vi "Swoish Grain Control.vi"() -> ()   [LabVIEW 2020]
uses:
  Type Defs/Motor Indicator.ctl
  Type Defs/Auto Params 1.ctl
  Type Defs/Numeric Big Up Down.ctl
  Type Defs/Auto Params 2.ctl
  Type Defs/Keyboard Button.ctl
  Type Defs/Email Config.ctl
  Type Defs/Alarm Limits.ctl
  Type Defs/Alarm Config.ctl
  Type Defs/PLC Coils.ctl
  Type Defs/Alarm Type.ctl
  <vilib>/Utility/miscctls.llb/LVPositionTypeDef.ctl
  Type Defs/Motor Pop-up Config Type Def.ctl
  Type Defs/Motors Type Def.ctl
  Type Defs/Motor Type Type Def.ctl
  Type Defs/Pop-up Corner Type Def.ctl
  Type Defs/Motor Data.ctl
  Type Defs/Info Config.ctl
  Type Defs/Modbus Mode.ctl
  Type Defs/HMI Coils.ctl
  Type Defs/Bin Indicator Type Def.ctl
  Type Defs/PLC Registers.ctl
  Type Defs/HMI Registers.ctl
  620634fb-1add-4c8b-beea-12df023673e0.vi
  142f28d0-f634-4b64-9fd9-03d418606ab8.vi
  <vilib>/httpClient/POSTBuffer.vi
  <vilib>/Comparison/Equal/Equal Functor/Equal Functor.lvclass
  <vilib>/httpClient/LabVIEWHTTPClient.lvlib
panel:
  in  "Array":u16[](array[slide])=[16055, 1251, 4170, 1460] scale=0.0..49000.0
  out "U-Trough":bool
  in  "Auto Mode Debug":bool
  in  "Exit":bool
  in  "Bin Levels Debug":u16[](array[numeric])
  out "Bin Levels":u16[](array[numeric])=[16055, 1251, 4170, 1460]
  in  "debug":bool
  in  "Alarms":T1[](array[typedef])=[{"PLC Coil"=enum."MC200_PLC_Estop_Main", "Alarm Type"=enum."Emergency", "Message"="The E-Stop on the main electrical enclosure was pushed.", "Shutdown"=TRUE, "Send Email"=TRUE}, {"PLC Coil"=enum."MC201_PLC_Estop_GSI", "Alarm Type"=enum."Emergency", "Message"="The E-Stop located on the GSI enclosure was pushed.", "Shutdown"=TRUE, "Send Email"=TRUE}, {"PLC Coil"=enum."MC202_PLC_Estop_Dryer", "Alarm Type"=enum."Emergency", "Message"="The E-Stop located at the Dryer was pushed.", "Shutdown"=TRUE, "Send Email"=TRUE}, {"PLC Coil"=enum."MC240_PLC_WS_Drag_OL", "Alarm Type"=enum."Warning", "Message"="Wet Silo Drag OVERLOAD.", "Shutdown"=FALSE, "Send Email"=TRUE}, {"PLC Coil"=enum."MC241_PLC_WB_Drag_OL", "Alarm Type"=enum."Warning", "Message"="Wet Bin Drag OVERLOAD.", "Shutdown"=FALSE, "Send Email"=TRUE}, {"PLC Coil"=enum."MC242_PLC_WS_Fan_OL", "Alarm Type"=enum."Warning", "Message"="Wet Silo Fan OVERLOAD.", "Shutdown"=FALSE, "Send Email"=TRUE}, {"PLC Coil"=enum."MC243_PLC_WB_Fan_OL", "Alarm Type"=enum."Warning", "Message"="Wet Bin Fan OVERLOAD.", "Shutdown"=FALSE, "Send Email"=TRUE}, {"PLC Coil"=enum."MC244_PLC_Dryr_Drag_OL", "Alarm Type"=enum."Warning", "Message"="Dryer Drag OVERLOAD.", "Shutdown"=FALSE, "Send Email"=TRUE}, {"PLC Coil"=enum."MC245_PLC_Dryr_Fan_OL", "Alarm Type"=enum."Warning", "Message"="Dryer Fan OVERLOAD.", "Shutdown"=FALSE, "Send Email"=TRUE}, {"PLC Coil"=enum."MC246_PLC_DB_Fan_Alm", "Alarm Type"=enum."Warning", "Message"="Dry Bin Fan VFD FAULT.", "Shutdown"=FALSE, "Send Email"=TRUE}, {"PLC Coil"=enum."MC247_PLC_DB_Drag_Alm", "Alarm Type"=enum."Warning", "Message"="Dry Bin Drag VFD FAULT.", "Shutdown"=FALSE, "Send Email"=TRUE}, {"PLC Coil"=enum."MC248_PLC_DB_Tp_Fd_Alm", "Alarm Type"=enum."Warning", "Message"="Dry Bin Top Feed VFD FAULT.", "Shutdown"=FALSE, "Send Email"=TRUE}, {"PLC Coil"=enum."MC249_PLC_U_Trough_Alm", "Alarm Type"=enum."Warning", "Message"="U-Trough VFD FAULT.", "Shutdown"=FALSE, "Send Email"=TRUE}, {"PLC Coil"=enum."MC250_PLC_Leg_Alm", "Alarm Type"=enum."Warning", "Message"="Leg VFD FAULT.", "Shutdown"=FALSE, "Send Email"=TRUE}, {"PLC Coil"=enum."MC261_PLC_Dryer_HI_Alm", "Alarm Type"=enum."Emergency", "Message"="The Dryer High Alarm limit switch has tripped.", "Shutdown"=TRUE, "Send Email"=TRUE}, {"PLC Coil"=enum."MC262_PLC_Dryr_Bin_Full", "Alarm Type"=enum."Warning", "Message"="The Dryer Bin Full limit switch has tripped.", "Shutdown"=FALSE, "Send Email"=TRUE}, {"PLC Coil"=enum."MC263_PLC_DB_HI_Alm", "Alarm Type"=enum."Warning", "Message"="The Dry Bin High Alarm limit switch has tripped.", "Shutdown"=FALSE, "Send Email"=TRUE}, {"PLC Coil"=enum."MC270_PLC_WS_Limit", "Alarm Type"=enum."Warning", "Message"="The Wet Silo has reached the level sensor limit.", "Shutdown"=FALSE, "Send Email"=TRUE}, {"PLC Coil"=enum."MC271_PLC_WB_Limit", "Alarm Type"=enum."Warning", "Message"="The Wet Bin has reached the level sensor limit.", "Shutdown"=FALSE, "Send Email"=TRUE}, {"PLC Coil"=enum."MC272_PLC_Dryr_Bin_Lim", "Alarm Type"=enum."Warning", "Message"="The Dryer Bin has reached the level sensor limit.", "Shutdown"=FALSE, "Send Email"=TRUE}, {"PLC Coil"=enum."MC273_PLC_DB_Limit", "Alarm Type"=enum."Warning", "Message"="The Dry Bin has reached the level sensor limit.", "Shutdown"=FALSE, "Send Email"=TRUE}, {"PLC Coil"=enum."MC274_PLC_Auto_Leg_Dry", "Alarm Type"=enum."Warning", "Message"="The Leg ran dry.  The Wet Bin or Silo may have run out of grain.", "Shutdown"=FALSE, "Send Email"=TRUE}, {"PLC Coil"=enum."MC280_Auto_Error_0", "Alarm Type"=enum."Warning", "Message"="While in Auto Mode, the Leg should have turned on, but didn't.", "Shutdown"=FALSE, "Send Email"=TRUE}, {"PLC Coil"=enum."MC281_Auto_Error_1", "Alarm Type"=enum."Warning", "Message"="While in Auto Mode, the Leg should have turned off, but didn't.", "Shutdown"=FALSE, "Send Email"=TRUE}, {"PLC Coil"=enum."MC282_Auto_Error_2", "Alarm Type"=enum."Warning", "Message"="While in Auto Mode, the Wet Bin Drag should have turned on, but didn't.", "Shutdown"=FALSE, "Send Email"=TRUE}, {"PLC Coil"=enum."MC283_Auto_Error_3", "Alarm Type"=enum."Warning", "Message"="While in Auto Mode, the Wet Bin Drag should have turned off, but didn't.", "Shutdown"=FALSE, "Send Email"=TRUE}, {"PLC Coil"=enum."MC284_Auto_Error_4", "Alarm Type"=enum."Warning", "Message"="While in Auto Mode, the Wet Silo Drag should have turned on, but didn't.", "Shutdown"=FALSE, "Send Email"=TRUE}, {"PLC Coil"=enum."MC285_Auto_Error_5", "Alarm Type"=enum."Warning", "Message"="While in Auto Mode, the Wet Silo Drag should have turned off, but didn't.", "Shutdown"=FALSE, "Send Email"=TRUE}, {"PLC Coil"=enum."MC286_Auto_Error_6", "Alarm Type"=enum."Warning", "Message"="While in Auto Mode, the Dry Bin Top Feed should have turned on, but didn't.", "Shutdown"=FALSE, "Send Email"=TRUE}, {"PLC Coil"=enum."MC287_Auto_Error_7", "Alarm Type"=enum."Warning", "Message"="While in Auto Mode, the Dry Bin Top Feed should have turned off, but didn't.", "Shutdown"=FALSE, "Send Email"=TRUE}]
  out "Heartbeat IN":bool
  out "Coils OUT":bool[](array[boolean])
  out "Registers OUT":u16[](array[numeric])
  out "Heartbeat OUT":bool=TRUE
  out "Loop Stop":bool
  out "PLC Disconnected":string="PLC DISCONNECTED!!!"
  in  "Alarm Pop-up":enum32{"Page 1"}(tab)
  in  "Alarm Ok PB":bool
  out "Alarm Title":string="Saturday, October 2, 2021  --  4:51:25 PM"
  out "Alarm Message":string="Saturday, October 2, 2021  --  4:51:25 PM"
  in  "VFD Pop-up":enum32{"Page 1"}(tab)
  in  "VFD_-1":bool
  in  "VFD_-0.1":bool
  in  "VFD_+0.1":bool
  in  "VFD_+1":bool
  out "VFD_Speed":dbl caption="bu" format="%.1f"
  out "VFD_Fault":bool caption="Fault"
  out "VFD_Running":bool caption="Running"
  in  "VFD_Toggle":bool
  in  "VFD_CMD":dbl caption="bu" min=0.0 max=60.0 format="%.1f"
  in  "VFD_Title":string="Leg"
  in  "Settings Pop-up":enum32{"Page 1"}(tab)
  in  "Settings Tab":T4(tab)=enum."Alarm Emails"
  in  "Auto Params 1":T5={"Leg Dry Limit:"=0, "Wet Drag Select:"=5, "Wet Drag Delay:"=0, "Leg Runout:"=0, "Dryer Bin Max:"=0, "Dryer Bin Min:"=0}
  in  "Auto Params 2":T7 {"Top Fd Auto Spd:" format="%.1f"}
  in  "Alarm Limits":T8={"Wet Silo Limit:"=5, "Wet Bin Limit:"=0, "Dryer Bin Limit:"=0, "Dry Bin Limit:"=0}
  in  "Email Config":T9[](array[typedef])=[{"Email"="garrett.tetil@gmail.com", "Enabled"=TRUE}, {"Email"="scott@myerselectricllc.com", "Enabled"=FALSE}, {"Email"="9896706221@txt.att.net", "Enabled"=TRUE}]
  in  "Settings Cancel PB":bool
  in  "Settings Ok PB":bool
  out "Auto Param Title":string="Settings"
  out "Keyboard PB":T10
  in  "Info Pop-up":enum32{"Page 1"}(tab)
  in  "Info Cancel PB":bool
  in  "Info Ok PB":bool
  out "Info Title":string="ATTENTION"
  out "Info Message":string="This will stop Auto Mode, and turn off all augers and drags."
  out "Motor_Sel (Round)":T11=TRUE
  out "Motor_Sel (Square)":bool
  in  "Motor Pop-up":enum32{"Page 1"}(tab)
  out "Motor_Overload":bool caption="Overload"
  out "Motor_Running":bool caption="Running"
  in  "Motor_Toggle":bool
  in  "Motor_Title":string="Wet Silo\nFan"
  in  "Main Tab":enum32{"Page 1"}(tab)
  in  "Reset Leg Dry PB":bool
  out "Leg Dry Run":bool
  out "DB Tp Fd Amps":dbl caption="bushel" format="%.1f A"
  out "Dryer Chute Open":bool
  out "Leg_Amps":dbl caption="bushel" format="%.1f A"
  out "Dryer Bin Level Limit":bool
  out "Wet Bin Level Limit":bool
  out "Wet Silo Level Limit":bool
  out "Dry Bin Level Limit":bool
  out "Auto Mode":bool
  in  "Settings PB":bool
  out "Date/Time String":string="Thursday, November 11, 2021  --  7:42:53 PM"
  out "Dryer Full":bool
  out "Dryer Bin Full":bool
  out "Dryer High Alarm":bool
  out "Dryer Feed":bool
  out "Dry Bin High Alarm":bool
  in  "Shutdown":bool
  in  "Auto/Manual PB":bool
  out "E-Stop (Dryer)":bool
  out "E-Stop (GSI)":bool
  out "E-Stop (Main)":bool
  out "WB_Numeric":u16=4170 caption="bushel"
  out "WS_Numeric":u16=1460 caption="bushel"
  out "Dryer_Numeric":u16=1251 caption="bushel"
  out "DB_Numeric":u16=16055 caption="bushel"
  out "DB_Scale":bool
  out "DB_Background":bool=TRUE
  out "DB_Fan":T11
  out "DB_Drag":T11
  out "Dryer_Fan":T11
  out "Dryer_Drag":T11
  out "WB_Fan":T11
  out "WS_Fan":T11
  out "WS_Drag":T11
  out "WB_Drag":T11
  out "Leg":bool
  out "DB_Top_Feed":bool
  out "Dryer_Scale":bool
  out "Dryer_Background":bool=TRUE
  out "WB_Scale":bool
  out "WB_Background":bool=TRUE
  out "WS_Scale":bool
  out "WS_Background":bool=TRUE
  # "Order dictates priority.\nMAKE VALUES DEFAULT!"
  # "Hz"
  # "Setpoint"
  # "Hz"
  # "Emails:"
  # "Enabled:"
  # "DRY BIN"
  # "WET SILO"
  # "DRY BIN\nTOP FEED"
  # "CONTROL\nROOM"
  # "LEG"
  # "DRYER /\nDRYER BIN"
  # "WET BIN"
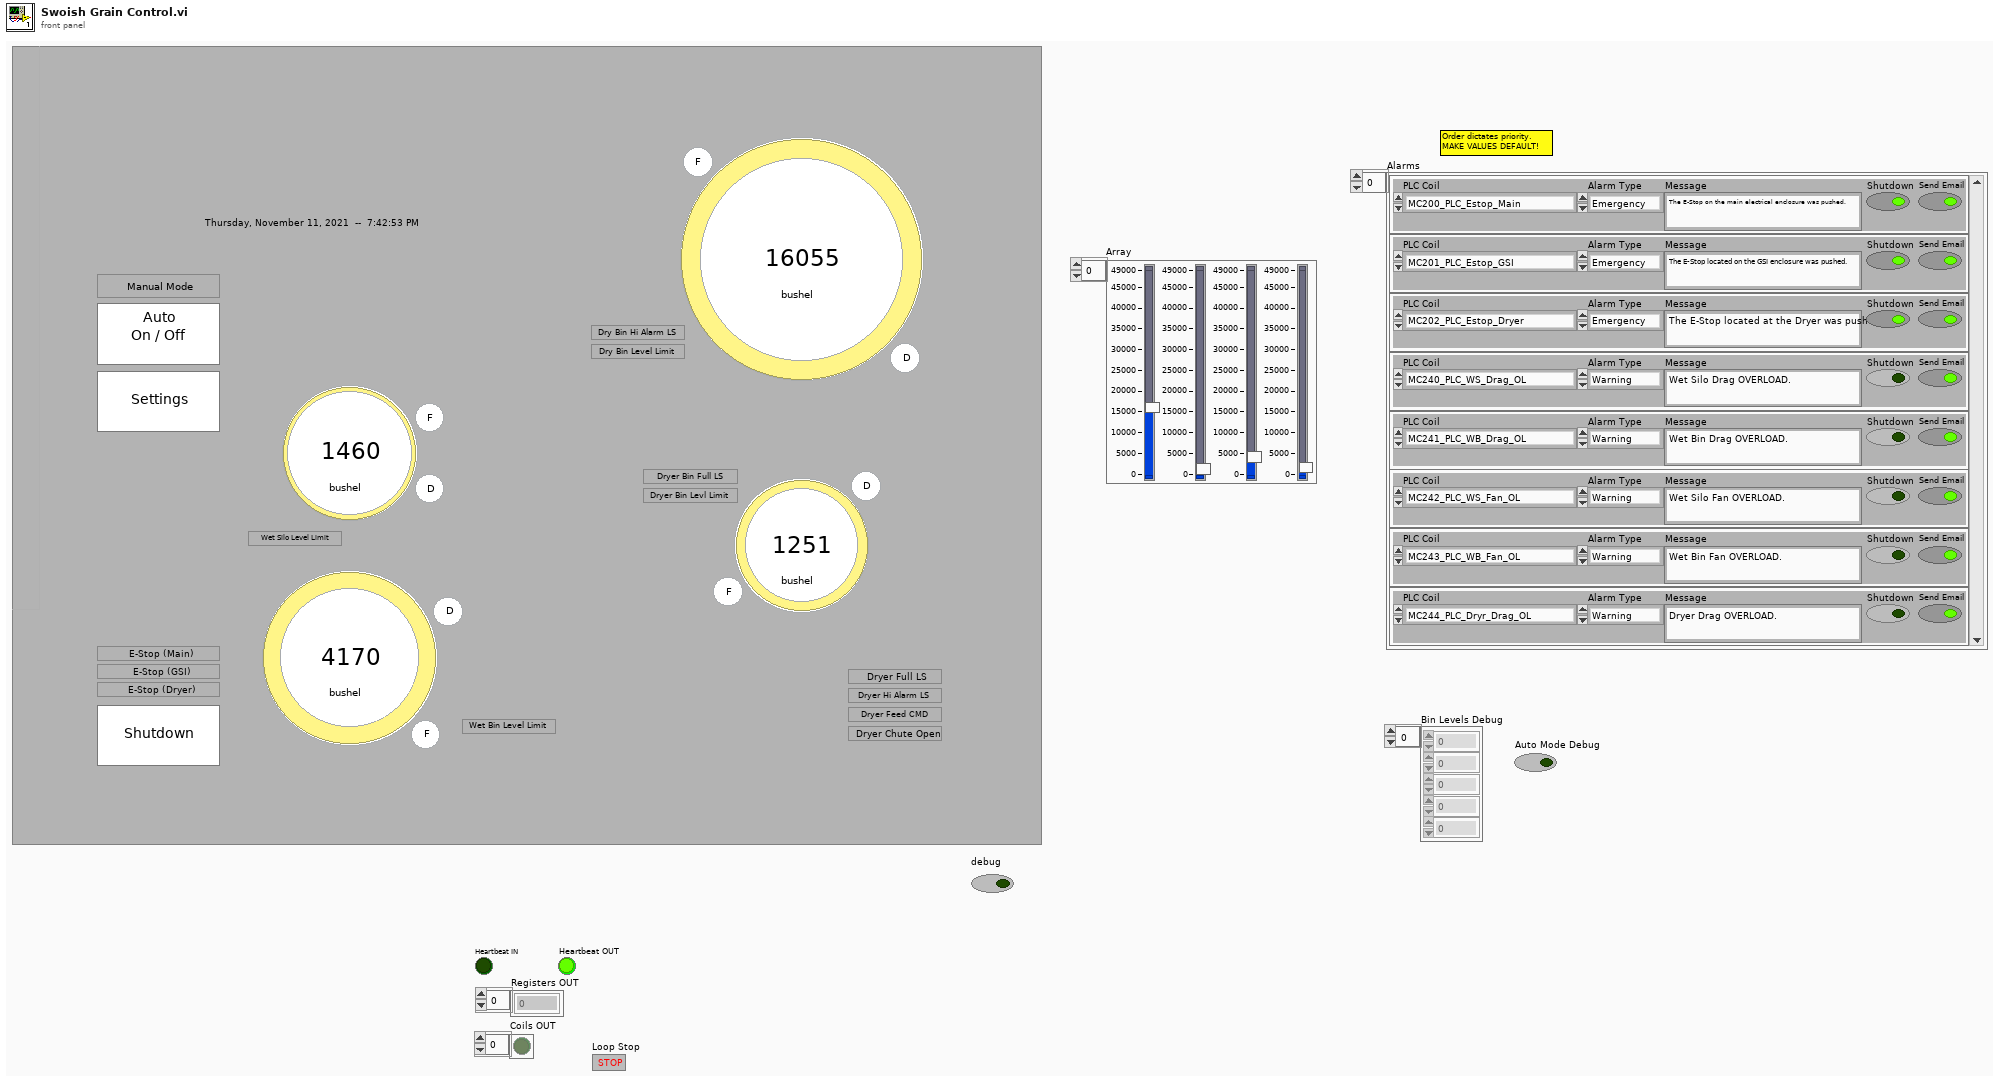
[diagram p1: front panel]
types:
  T1 = typedef "Alarm Config.ctl" = cluster{"PLC Coil":T2, "Alarm Type":T3, "Message":string, "Shutdown":bool, "Send Email":bool}
  T2 = typedef "PLC Coils.ctl" = enum16{"MC200_PLC_Estop_Main", "MC201_PLC_Estop_GSI", "MC202_PLC_Estop_Dryer", "MC203_PLC_Auto_Mode", "MC204", "MC205", "MC206", "MC207", "MC208", "MC209", "MC210", "MC211", "MC212", "MC213", "MC214", "MC215", "MC216", "MC217", "MC218", "MC219", "MC220_PLC_WS_Drag_ON", "MC221_PLC_WB_Drag_ON", "MC222_PLC_WS_Fan_ON", "MC223_PLC_WB_Fan_ON", "MC224_PLC_Dryr_Drag_ON", "MC225_PLC_Dryr_Fan_ON", "MC226", "MC227", "MC228", "MC229", "MC230", "MC231", "MC232", "MC233", "MC234", "MC235", "MC236", "MC237", "MC238", "MC239", "MC240_PLC_WS_Drag_OL", "MC241_PLC_WB_Drag_OL", "MC242_PLC_WS_Fan_OL", "MC243_PLC_WB_Fan_OL", "MC244_PLC_Dryr_Drag_OL", "MC245_PLC_Dryr_Fan_OL", "MC246_PLC_DB_Fan_Alm", "MC247_PLC_DB_Drag_Alm", "MC248_PLC_DB_Tp_Fd_Alm", "MC249_PLC_U_Trough_Alm", "MC250_PLC_Leg_Alm", "MC251", "MC252", "MC253", "MC254", "MC255", "MC256", "MC257", "MC258", "MC259", "MC260_PLC_Dryer_Full", "MC261_PLC_Dryer_HI_Alm", "MC262_PLC_Dryr_Bin_Full", "MC263_PLC_DB_HI_Alm", "MC264_PLC_Dryer_Chute", "MC265_PLC_Dryer_Feed", "MC266", "MC267", "MC268", "MC269", "MC270_PLC_WS_Limit", "MC271_PLC_WB_Limit", "MC272_PLC_Dryr_Bin_Lim", "MC273_PLC_DB_Limit", "MC274_PLC_Auto_Leg_Dry", "MC275", "MC276", "MC277", "MC278", "MC279", "MC280_Auto_Error_0", "MC281_Auto_Error_1", "MC282_Auto_Error_2", "MC283_Auto_Error_3", "MC284_Auto_Error_4", "MC285_Auto_Error_5", "MC286_Auto_Error_6", "MC287_Auto_Error_7", "MC288_Auto_Error_8", "MC289_Auto_Error_9"}
  T3 = typedef "Alarm Type.ctl" = enum16{"Warning", "Emergency"}
  T4 = enum32{"Auto Params", "Alarm Limits", "Alarm Emails"}
  T5 = typedef "Auto Params 1.ctl" = cluster{"Leg Dry Limit:":T6, "Wet Drag Select:":T6, "Wet Drag Delay:":T6, "Leg Runout:":T6, "Dryer Bin Max:":T6, "Dryer Bin Min:":T6}
  T6 = typedef "Numeric Big Up Down.ctl" = u16
  T7 = typedef "Auto Params 2.ctl" = cluster{"Top Fd Auto Spd:":dbl}
  T8 = typedef "Alarm Limits.ctl" = cluster{"Wet Silo Limit:":T6, "Wet Bin Limit:":T6, "Dryer Bin Limit:":T6, "Dry Bin Limit:":T6}
  T9 = typedef "Email Config.ctl" = cluster{"Email":string, "Enabled":bool}
  T10 = typedef "Keyboard Button.ctl" = bool
  T11 = typedef "Motor Indicator.ctl" = bool
  T12 = typedef "Info Config.ctl" = cluster{"Title":string, "Message":string, "Next State":string}
  T13 = typedef "Motor Data.ctl" = cluster{"Running":bool, "OL/Fault":bool, "VFD Speed":dbl, "VFD CMD":dbl}
  T14 = typedef "LVPositionTypeDef.ctl" = cluster{"Left":i32, "Top":i32}
  T15 = typedef "Motor Pop-up Config Type Def.ctl" = cluster{"Motor/VFD":T16, "Motor Type":T17, "Pop-up Corner":T18}
  T16 = typedef "Motors Type Def.ctl" = enum16{"WS_Drag", "WB_Drag", "WS_Fan", "WB_Fan", "Dryer_Drag", "Dryer_Fan", "DB_Fan", "DB_Drag", "DB_Top_Feed", "U-Trough", "Leg"}
  T17 = typedef "Motor Type Type Def.ctl" = enum16{"MS", "VFD"}
  T18 = typedef "Pop-up Corner Type Def.ctl" = enum16{"Top Left", "Top Right", "Bottom Left", "Bottom Right"}
  T19 = typedef "LabVIEWHTTPClient.lvlib/ClientHandle.ctl" = refnum<k1>
  T20 = cluster{"debug":bool, "Error":errorcluster, "Pop-up Config":T15, "Motor Descriptions":string[], "Pop-up Offset":T14, "Default Offset":T14, "Selected Motor Ref":refnum<vi>, "Motor Toggle":bool, "PLC Coils":bool[], "PLC Regs":u16[], "Motor Refs":refnum<vi>[], "Motor Data":T13[], "VFD_CMD":dbl, "Alarms":T1[], "Prev Alarm States":bool[], "Active Alarm Config":T1, "Active Alarm":bool, "Info Config":T12, "Params Open":bool, "Heartbeat Timer":u32, "Connected":bool, "Mode Toggle":bool, "Email Config":T9[], "Email Config Path":path}
  T21 = typedef "Modbus Mode.ctl" = enum16{"Init", "Read", "Write Coil", "Write Reg", "Param Read", "Param Write", "Close"}
  T22 = typedef "HMI Coils.ctl" = enum16{"MC100_HMI_WS_Drag_PB", "MC101_HMI_WB_Drag_PB", "MC102_HMI_WS_Fan_PB", "MC103_HMI_WB_Fan_PB", "MC104_HMI_Dryr_Drag_PB", "MC105_HMI_Dryr_Fan_PB", "MC106_HMI_DB_Fan_PB", "MC107_HMI_DB_Drag_PB", "MC108_HMI_DB_Top_Feed_PB", "MC109_HMI_U-Trough_PB", "MC110_HMI_Leg_PB", "MC111", "MC112", "MC113", "MC114", "MC115", "MC116", "MC117", "MC118", "MC119", "MC120_HMI_Shutdown", "MC121_HMI_Mode_Toggle", "MC122_HMI_Reset_Leg_Dry", "MC123"}
  T23 = cluster{"Running":bool, "OL/Fault":bool, "VFD Speed":dbl, "VFD CMD":dbl}
  T24 = typedef "Bin Indicator Type Def.ctl" = cluster{"Scale":refnum<vi>, "Background":refnum<vi>, "Numeric":refnum<vi>, "Bin Max":u16}
  T25 = enum8{"Enabled", "Disabled", "Disabled and Grayed Out"}
  T26 = typedef "PLC Registers.ctl" = enum16{"MHR200_PLC_DB_Fan_Spd", "MHR201_PLC_DB_Drag_Spd", "MHR202_PLC_DB_Tp_Fd_Spd", "MHR203_PLC_U_Trough_Spd", "MHR204_PLC_Leg_Spd", "MHR205_PLC_DB_Fan_ON", "MHR206_PLC_DB_Drag_ON", "MHR207_PLC_DB_Tp_Fd_ON", "MHR208_PLC_U_Trough_ON", "MHR209_PLC_Leg_ON", "MHR210_PLC_DB_Fan_CMD", "MHR211_PLC_DB_Drag_CMD", "MHR212_PLC_DB_Tp_Fd_CMD", "MHR213_PLC_U_Trough_CMD", "MHR214_PLC_Leg_CMD", "MHR215_PLC_DB_Fan_Flt", "MHR216_PLC_DB_Drag_Flt", "MHR217_PLC_DB_Tp_Fd_Flt", "MHR218_PLC_U_Trough_Flt", "MHR219_PLC_Leg_Flt", "MHR220_PLC_DB_Level", "MHR221_PLC_WB_Level", "MHR222_PLC_WS_Level", "MHR223_PLC_Dryr_Bin_Level", "MHR224_PLC_Leg_Amps", "MHR225_PLC_DB_Tp_Fd_Amps"}
  T27 = typedef "HMI Registers.ctl" = enum16{"MHR100_HMI_DB_Fan_CMD", "MHR101_HMI_DB_Drag_CMD", "MHR102_HMI_DB_TF_CMD", "MHR103_HMI_U_Trough_CMD", "MHR104_HMI_Leg_CMD"}
  T28 = cluster{"Running":bool, "OL/Fault":bool, "VFD Speed":dbl, "VFD CMD":dbl}[]
  T29 = cluster{"[0]":u16, "[1]":u16, "[2]":u16, "[3]":u16, "[4]":u16, "[5]":u16}
  T30 = cluster{"[0]":u16, "[1]":u16, "[2]":u16, "[3]":u16}
  T31 = enum32{"invalid app kind", "Development System", "Run Time System", "Student Edition", "Embedded LabVIEW", "Evaluation", "Custom"}
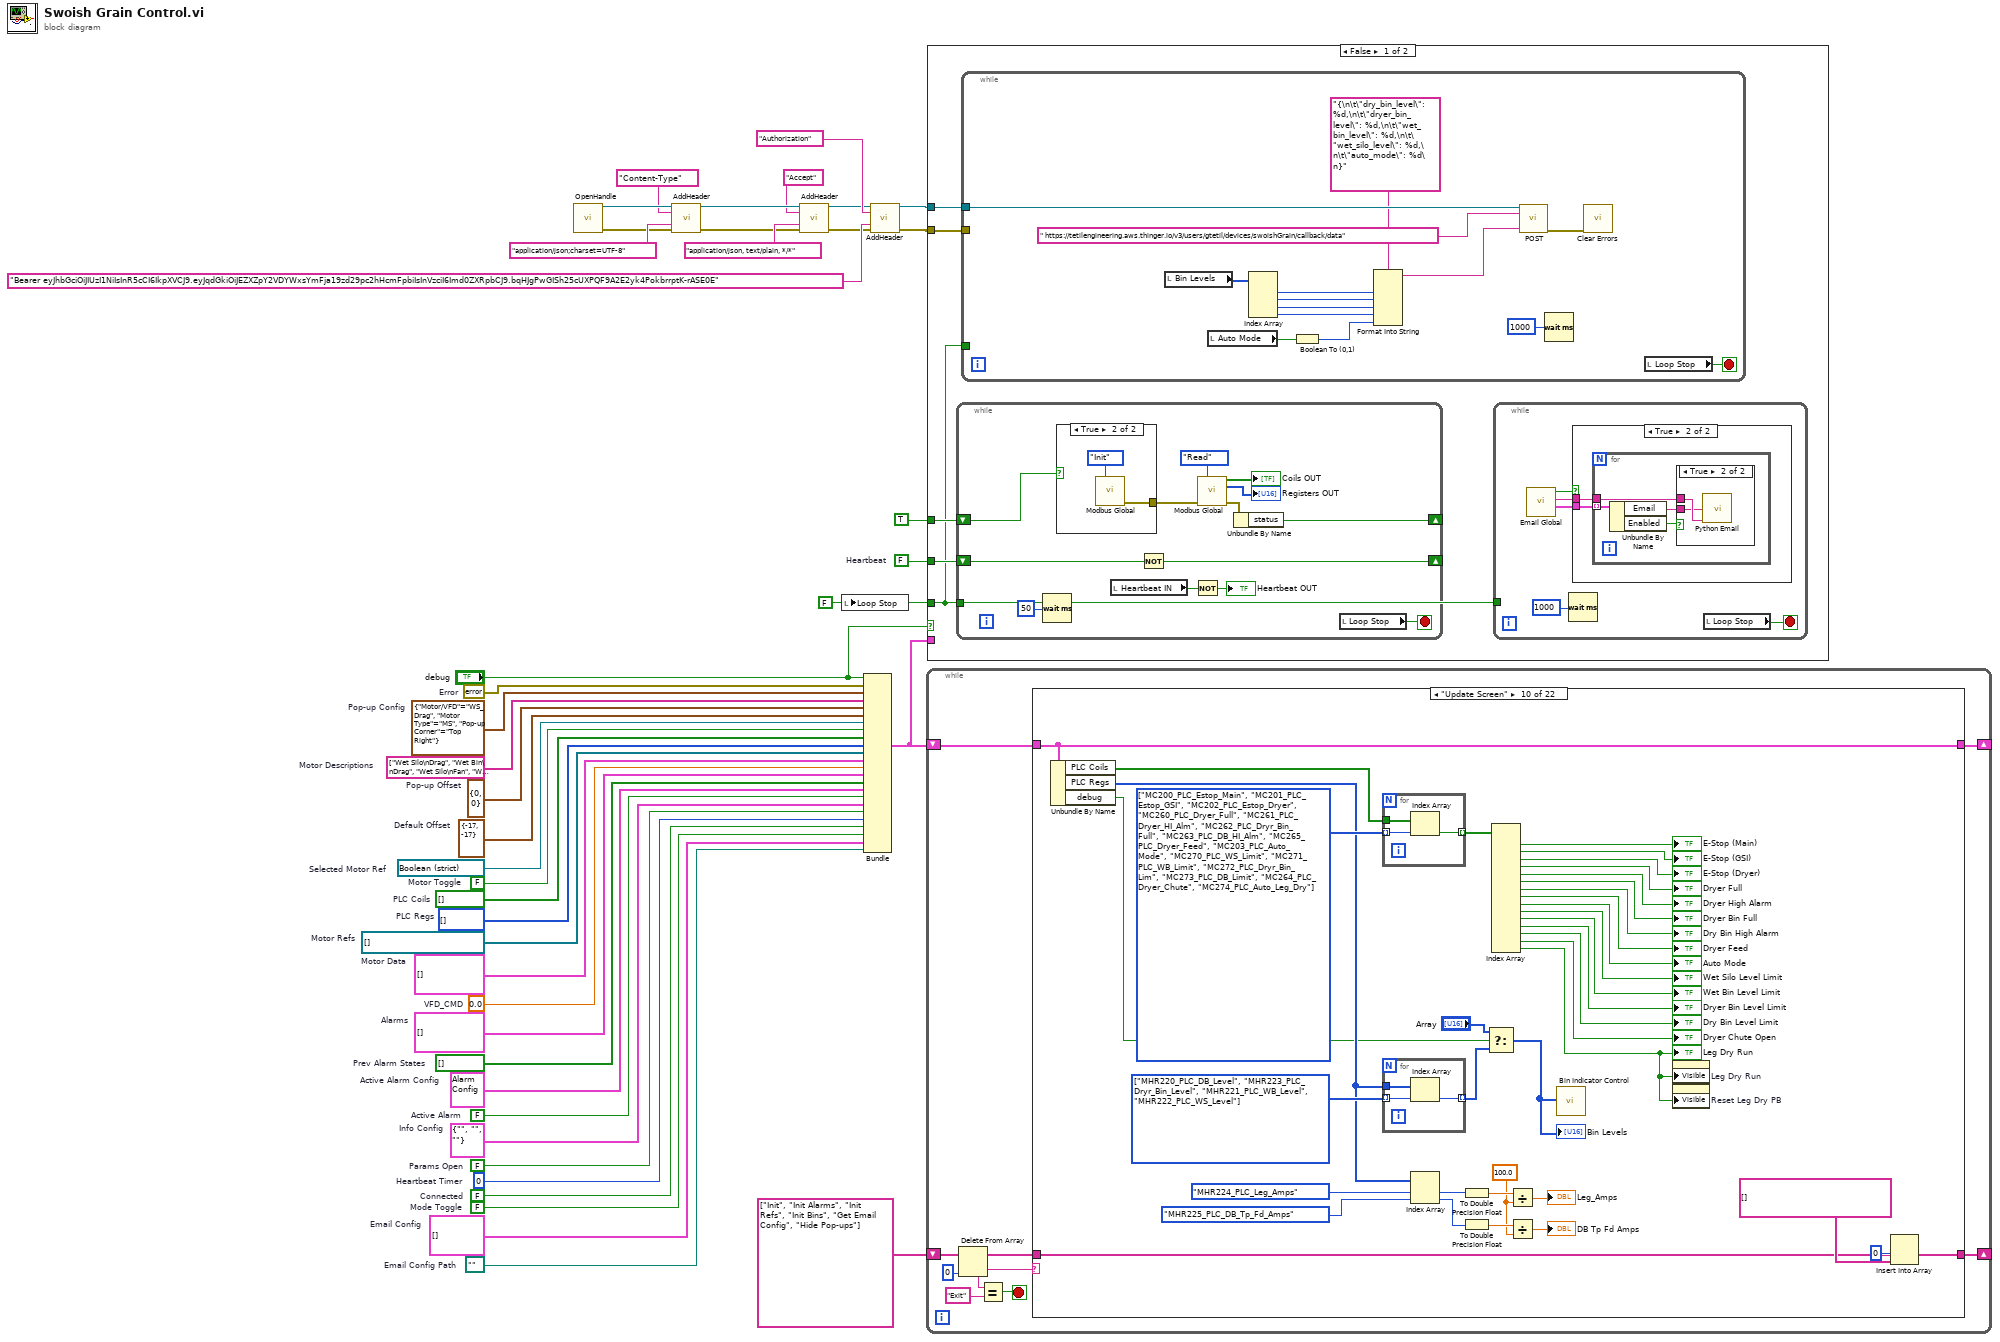
[diagram p0: block diagram]
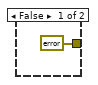
[diagram p2: hidden frame]
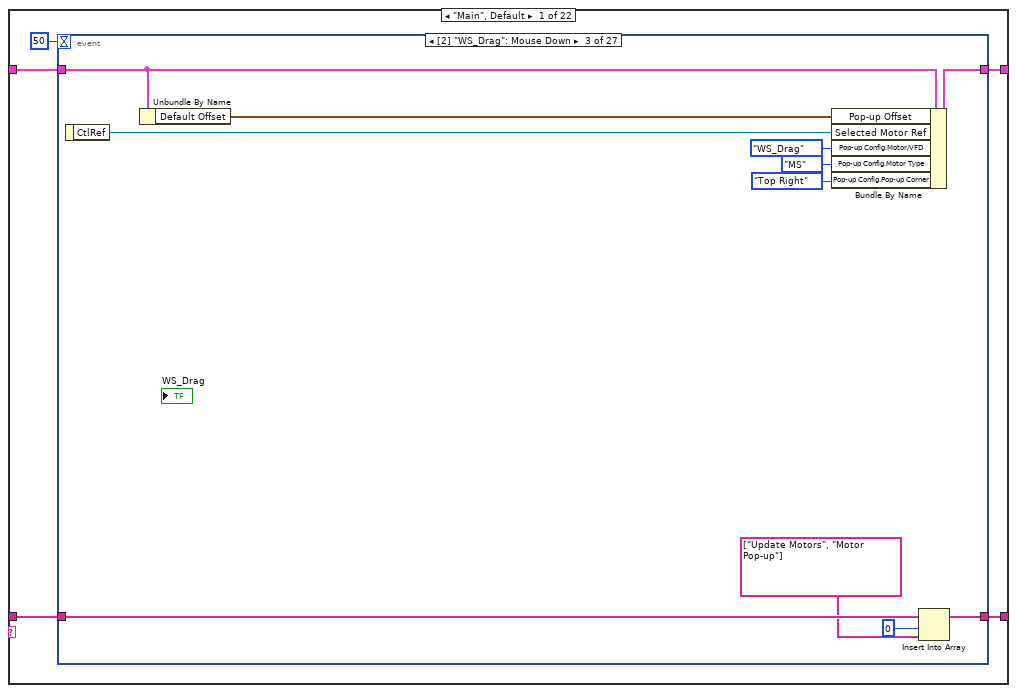
[diagram p6: hidden frame]
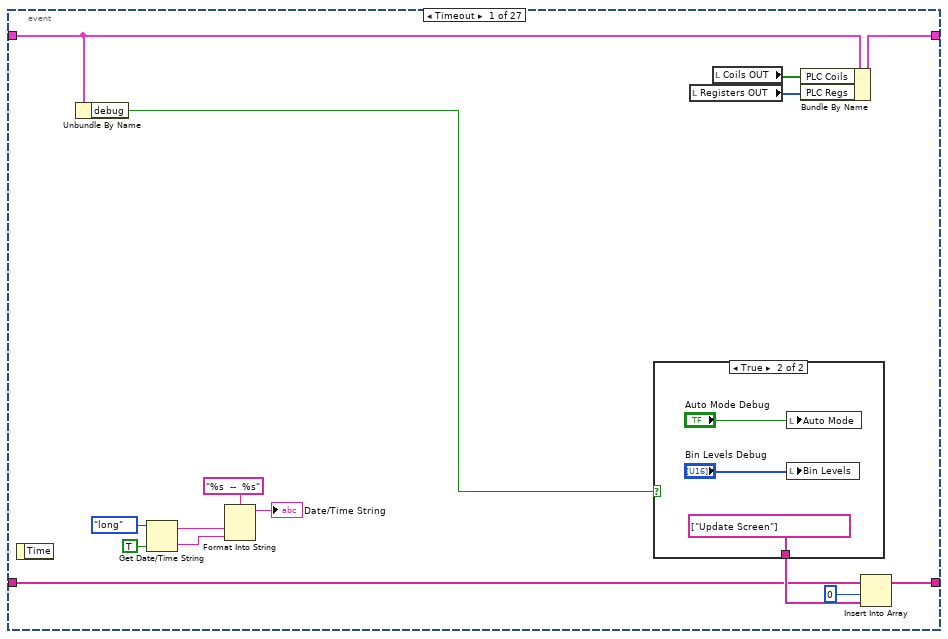
[diagram p7: hidden frame]
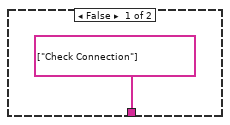
[diagram p8: hidden frame]
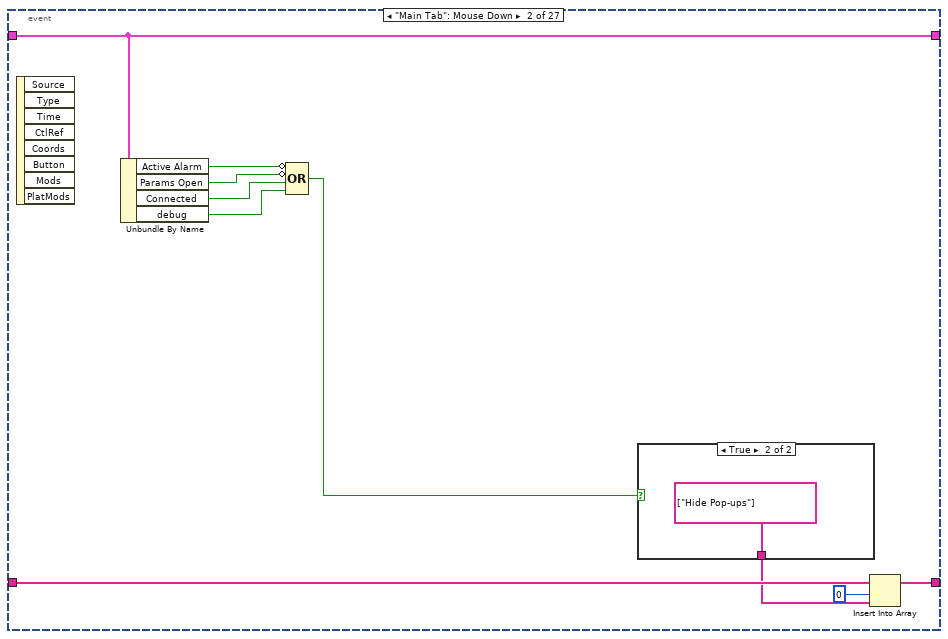
[diagram p9: hidden frame]
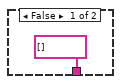
[diagram p10: hidden frame]
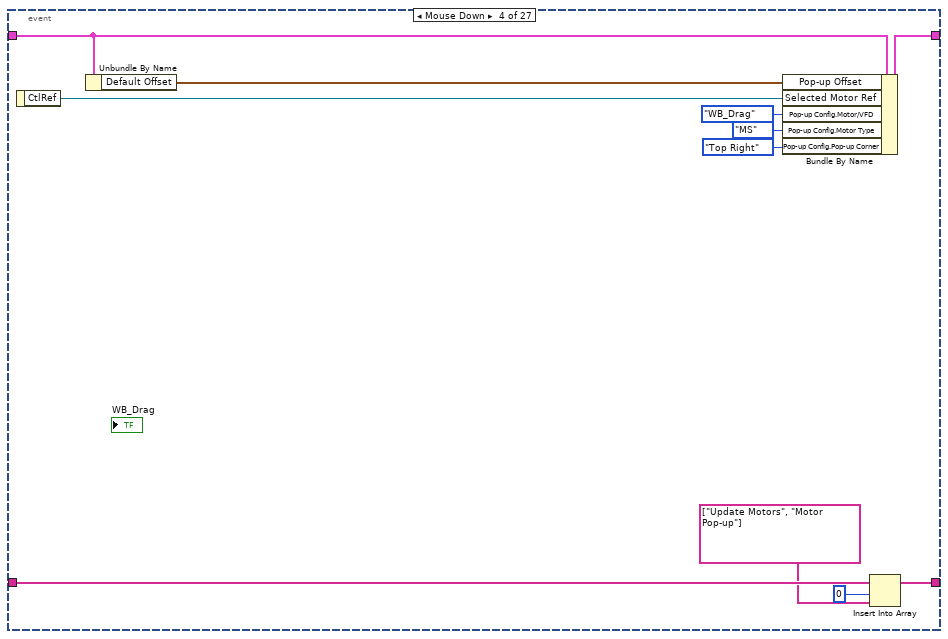
[diagram p11: hidden frame]
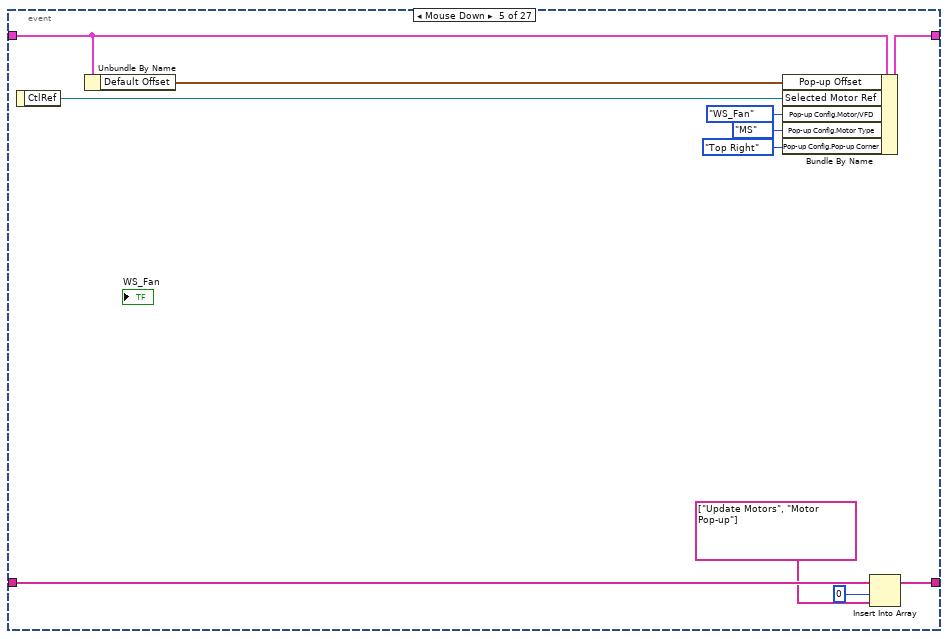
[diagram p12: hidden frame]
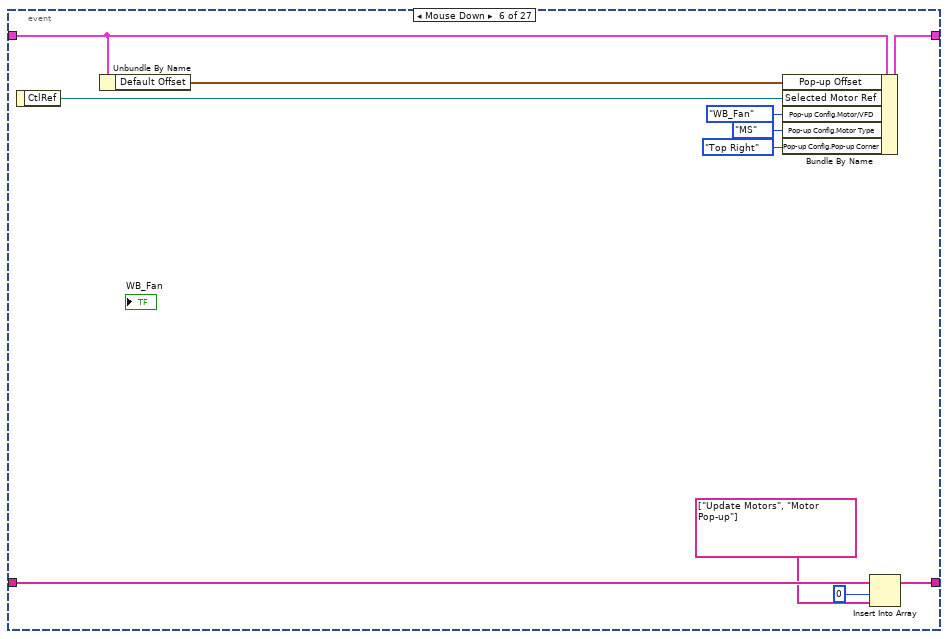
[diagram p13: hidden frame]
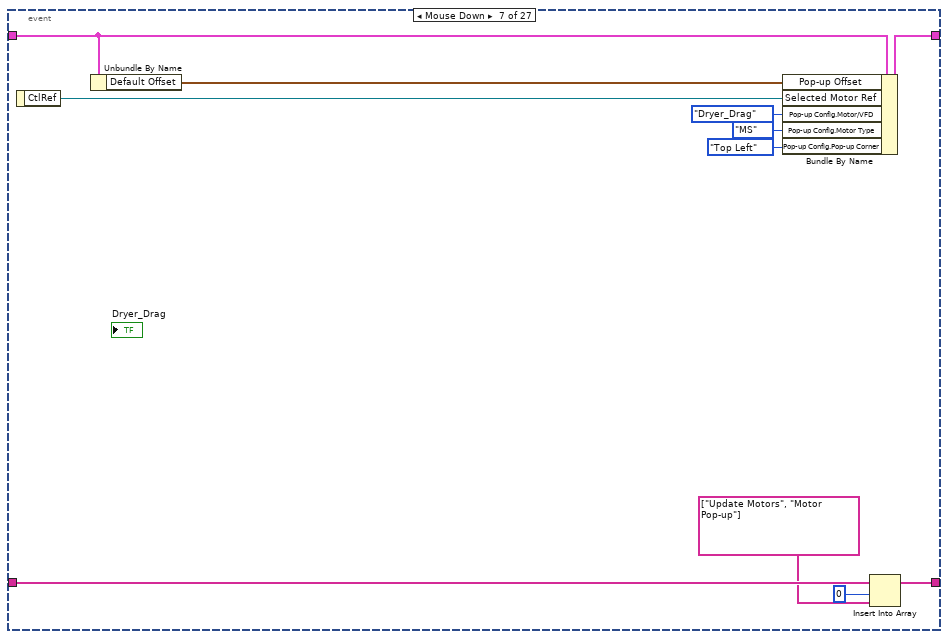
[diagram p14: hidden frame]
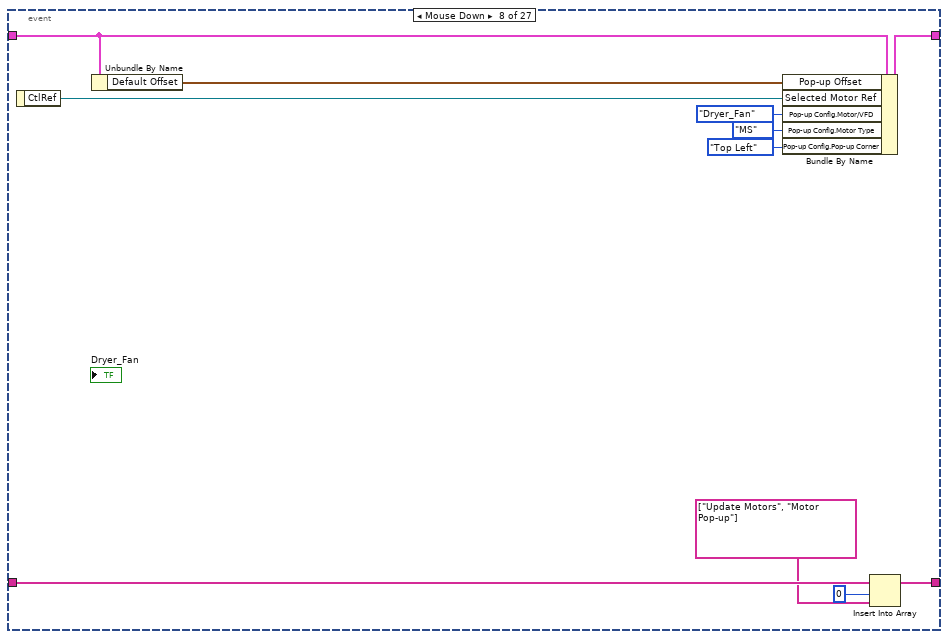
[diagram p15: hidden frame]
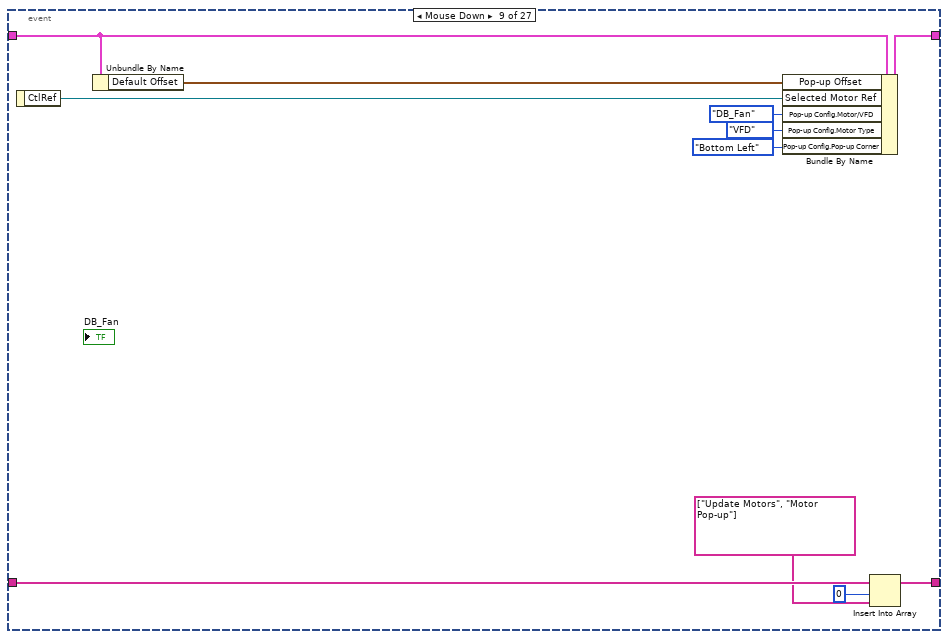
[diagram p16: hidden frame]
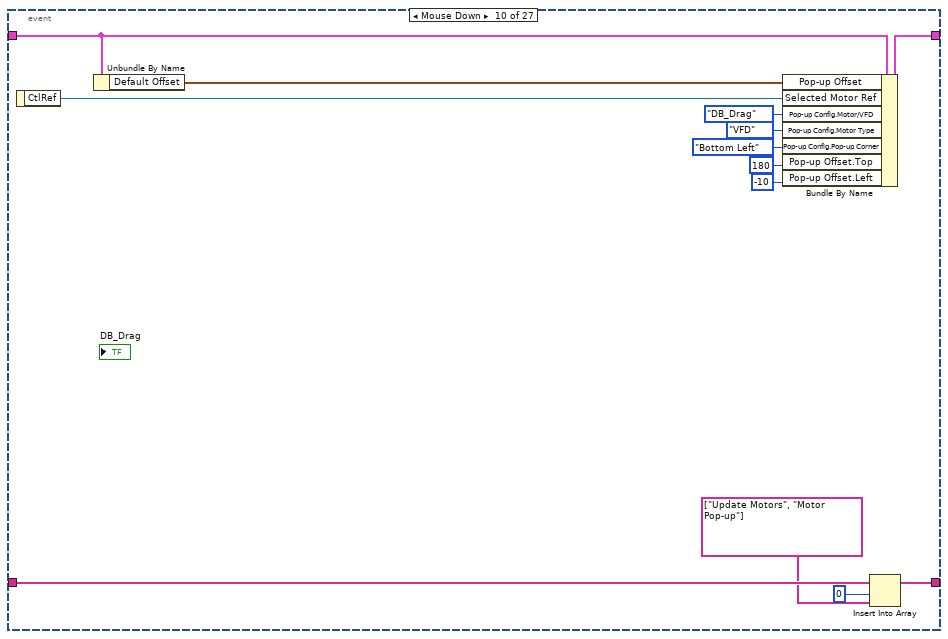
[diagram p17: hidden frame]
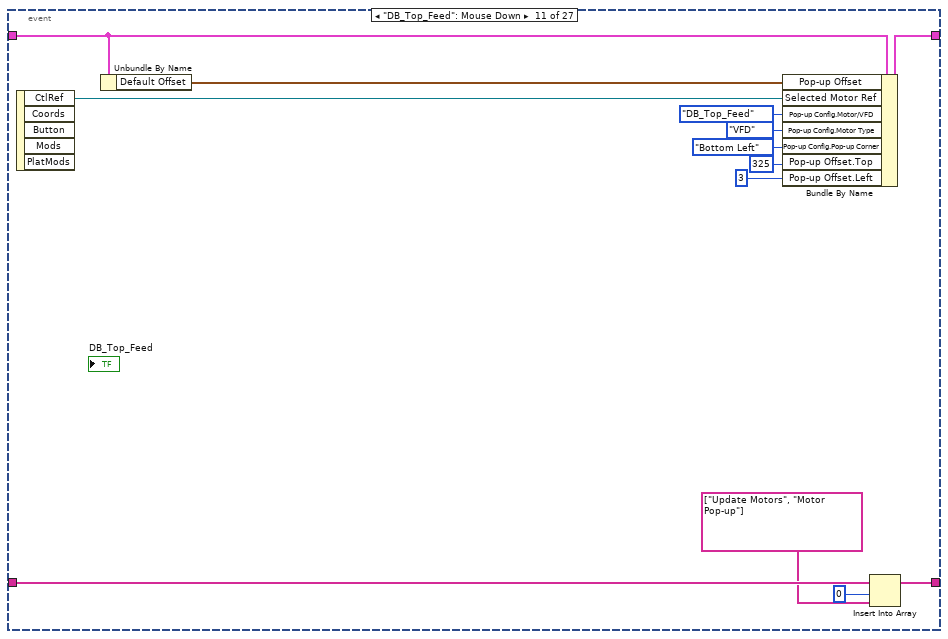
[diagram p18: hidden frame]
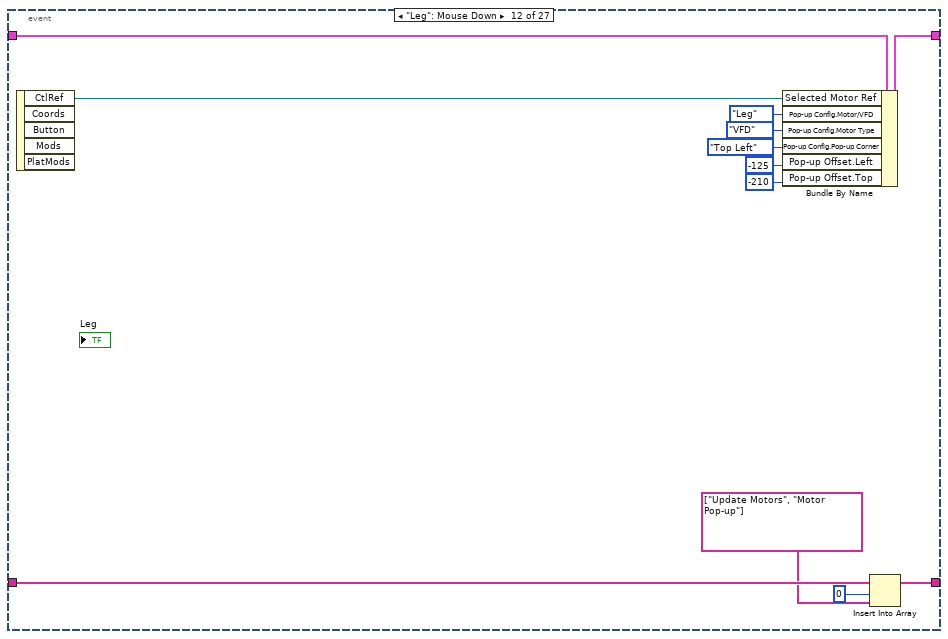
[diagram p19: hidden frame]
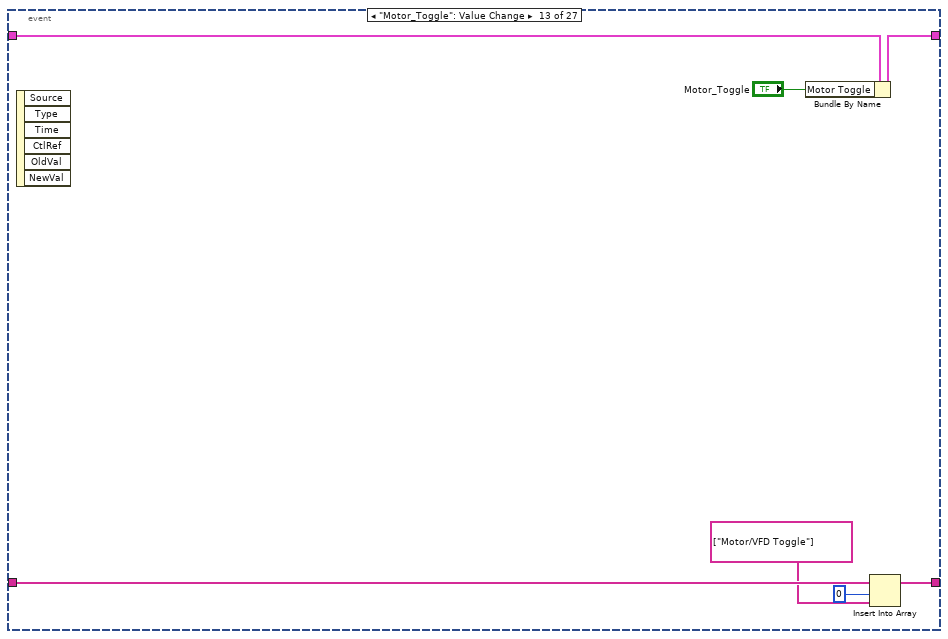
[diagram p20: hidden frame]
diagram:
  w18 = path ""  # Email Config Path
  w19 = T9[] []  # Email Config
  w20 = FALSE  # Mode Toggle
  w21 = FALSE  # Connected
  w23 = u32 0  # Heartbeat Timer
  w24 = FALSE  # Heartbeat
  w7 = FALSE ("Modbus Stop")
  w25 = FALSE  # Params Open
  w26 = T12 {"Title"="", "Message"="", "Next State"=""}  # Info Config
  w27 = FALSE  # Active Alarm
  w28 = T1 {"PLC Coil"=enum."MC200_PLC_Estop_Main", "Alarm Type"=enum."Warning", "Message"="", "Shutdown"=FALSE, "Send Email"=FALSE}  # Active Alarm Config
  w29 = bool[] []  # Prev Alarm States
  w30 = T1[] []  # Alarms
  w31 = 0.0  # VFD_CMD
  w32 = T13[] []  # Motor Data
  w33 = refnum<vi>[] []  # Motor Refs
  w34 = u16[] []  # PLC Regs
  w35 = bool[] []  # PLC Coils
  w36 = FALSE  # Motor Toggle
  w37 = T14 {"Left"=-17, "Top"=-17}  # Default Offset
  w38 = refnum<vi> refnum  # Selected Motor Ref
  w39 = T15 {"Motor/VFD"=enum."WS_Drag", "Motor Type"=enum."MS", "Pop-up Corner"=enum."Top Right"}  # Pop-up Config
  w41 = string[] ["Wet Silo\nDrag", "Wet Bin\nDrag", "Wet Silo\nFan", "Wet Bin\nFan", "Dryer\nDrag", "Dryer\nFan", "Dry Bin\nFan", "Dry Bin\nDrag", "Dry Bin\nTop Feed", "U-Trough", "Leg"]  # Motor Descriptions
  w40 = T14 {"Left"=0, "Top"=0}  # Pop-up Offset
  w42 = errorcluster {"status"=FALSE, "code"=0, "source"=""}  # Error
  n1 = call <vilib>:"OpenHandle.vi"() -> ("client handle out"=w17:T19, "error out"=w6:errorcluster)  [unwired: 14 in]
  n2 = call <vilib>:"AddHeader.vi"("client handle"=w17, "header"="Content-Type", "value"="application/json;charset=UTF-8", "error in (no error)"=w6) -> ("client handle out"=w11:T19, "error out"=w5:errorcluster)  [unwired: 10 in]
  n3 = call <vilib>:"AddHeader.vi"("client handle"=w11, "header"="Accept" ("value"), "value"="application/json, text/plain, */*", "error in (no error)"=w5) -> ("client handle out"=w10:T19, "error out"=w4:errorcluster)  [unwired: 10 in]
  n4 = local write "Loop Stop"(w7) -> ()
  n5 = Bundle("debug"="debug", "Error"=w42, "Pop-up Config"=w39, "Motor Descriptions"=w41, "Pop-up Offset"=w40, "Default Offset"=w37, "Selected Motor Ref"=w38, "Motor Toggle"=w36, "PLC Coils"=w35, "PLC Regs"=w34, "Motor Refs"=w33, "Motor Data"=w32, "VFD_CMD"=w31, "Alarms"=w30, "Prev Alarm States"=w29, "Active Alarm Config"=w28, "Active Alarm"=w27, "Info Config"=w26, "Params Open"=w25, "Heartbeat Timer"=w23, "Connected"=w21, "Mode Toggle"=w20, "Email Config"=w19, "Email Config Path"=w18) -> (w2:T20)  [unwired: 1 in]
  n6 = call <vilib>:"AddHeader.vi"("client handle"=w10, "header"="Authorization" ("value"), "value"="Bearer eyJhbGciOiJIUzI1NiIsInR5cCI6IkpXVCJ9.eyJqdGkiOiJEZXZpY2VDYWxsYmFja19zd29pc2hHcmFpbiIsInVzciI6Imd0ZXRpbCJ9.bqHJgPwGISh25cUXPQF9A2E2yk4PokbrrptK-rASE0E", "error in (no error)"=w4) -> ("client handle out"=w13:T19, "error out"=w3:errorcluster)  [unwired: 10 in]
  n7 = while {
    shift-right: [w47] -> _
    shift-left: w2 -> [w52]
    shift-right: [w48] -> _
    shift-left: string[] ["Init", "Init Alarms", "Init Refs", "Init Bins", "Get Email Config", "Hide Pop-ups"] -> [w51]
    stop <- w44 stop-if-true
    n8 = Delete From Array(array=w51, index=0) -> (deleted portion=w46:string, array with subset deleted=w49:string[])  [unwired: 1 in]
    n9 = Equal?(x=w46, y="Exit") -> (x = y?=w44:bool)
    n10 = case shown="\"Update Screen\"" w46 {
      tunnel: w52 -> [w57 w348 w357 w378 w412 w420 w429 w442 w480 w533 w556 w597 w615 w620 w633 w672 w700 w711 w734 w753 w764 w771]
      tunnel: w49 -> [w55 w350 w360 w381 w414 w426 w431 w451 w492 w535 w559 w584 w617 w624 w637 w680 w705 w713 w736 w755 w766 w774]
      tunnel: [w54 w349 w359 w380 w413 w425 w430 w435 w491 w534 w558 w599 w616 w623 w636 w679 w704 w712 w735 w754 w765 w773] -> w48
      tunnel: [w56 w348 w358 w379 w412 w421 w429 w443 w481 w533 w557 w598 w615 w620 w635 w673 w703 w711 w734 w753 w764 w771] -> w47
      frame "Main", Default {
        n11 = event shown="[2] \"WS_Drag\": Mouse Down" {
          selector: _ -> [_ _ _ _ _ _ _ _ _ _ _ _ _ _ _ _ _ _ _ _ _ _ _ _ _ _ _]
          dyn-events: _ -> [_ _ _ _ _ _ _ _ _ _ _ _ _ _ _ _ _ _ _ _ _ _ _ _ _ _ _]
          timeout: 50 -> [_ _ _ _ _ _ _ _ _ _ _ _ _ _ _ _ _ _ _ _ _ _ _ _ _ _ _]
          tunnel: w57 -> [w59 w82 w90 w102 w113 w124 w135 w146 w157 w170 w182 w197 w206 w213 w223 w247 w256 w264 w271 w282 w287 w291 w296 w310 w325 w333 w340]
          tunnel: [w62 w82 w95 w107 w118 w129 w140 w151 w162 w175 w188 w200 w205 w212 w231 w248 w256 w265 w272 w282 w287 w291 w296 w311 w325 w333 w340] -> w56
          tunnel: w55 -> [w69 w86 w99 w110 w121 w132 w143 w154 w165 w178 w191 w203 w210 w217 w235 w252 w260 w269 w276 w280 w286 w295 w300 w324 w329 w337 w344]
          tunnel: [w72 w85 w98 w109 w120 w131 w142 w153 w164 w177 w190 w202 w209 w216 w234 w251 w259 w268 w275 w285 w290 w294 w299 w323 w328 w336 w343] -> w54
          event Timeout {
            n12 = event-data() -> ()  [unwired: 1 in, 1 out]
            n13 = Unbundle By Name(w59) -> ("debug"=w58:bool)
            n14 = Get Date/Time String(date format (0)=enum16{"short", "long", "abbreviated"}."long", want seconds? (F)=TRUE) -> (date string=w67:string, time string=w66:string)  [unwired: 1 in]
            n15 = Format Into String(format string="%s  --  %s", w67, w66) -> (resulting string=→"Date/Time String":string)  [unwired: 2 in, 1 out]
            n16 = case shown="True" w58 {
              tunnel: [string[] ["Check Connection"] string[] ["Update Screen"]] -> w70
              frame False {
              }
              frame True {
                n17 = local write "Auto Mode"("Auto Mode Debug") -> ()
                n18 = local write "Bin Levels"("Bin Levels Debug") -> ()
              }
            }
            n19 = local read "Registers OUT"() -> (w60:u16[])
            n20 = local read "Coils OUT"() -> (w61:bool[])
            n21 = Bundle By Name(cluster=w59, "PLC Coils"=w61, "PLC Regs"=w60) -> (w62:T20)
            n22 = Insert Into Array(array=w69, index=0, new element=w70) -> (w72:string[])
          }
          event "Main Tab": Mouse Down {
            n23 = event-data() -> ()  [unwired: 1 in, 8 out]
            n24 = Unbundle By Name(w82) -> ("Active Alarm"=w81:bool, "Params Open"=w80:bool, "Connected"=w78:bool, "debug"=w77:bool)
            n25 = Compound Arithmetic op=OR(invert w81, invert w80, w78, w77) -> (w79:bool)
            n26 = case shown="True" w79 {
              tunnel: [string[] [] string[] ["Hide Pop-ups"]] -> w83
              frame False {
              }
              frame True {
              }
            }
            n27 = Insert Into Array(array=w86, index=0, new element=w83) -> (w85:string[])
          }
          event Mouse Down {
            n28 = event-data() -> ("CtlRef"=w91:refnum<vi>)  [unwired: 1 in]
            n29 = Unbundle By Name(w90) -> ("Default Offset"=w89:T14)
            n30 = Bundle By Name(cluster=w90, "Pop-up Offset"=w89, "Selected Motor Ref"=w91, "Pop-up Config.Motor/VFD"=Motors_Type_Def."WS_Drag" ("Pop-up Config.Motor"), "Pop-up Config.Motor Type"=Motor_Type_Type_Def."MS", "Pop-up Config.Pop-up Corner"=Pop-up_Corner_Type_Def."Top Right") -> (w95:T20)
            n31 = Insert Into Array(array=w99, index=0, new element=string[] ["Update Motors", "Motor Pop-up"]) -> (w98:string[])
          }
          event Mouse Down {
            n32 = event-data() -> ("CtlRef"=w103:refnum<vi>)  [unwired: 1 in]
            n33 = Unbundle By Name(w102) -> ("Default Offset"=w101:T14)
            n34 = Bundle By Name(cluster=w102, "Pop-up Offset"=w101, "Selected Motor Ref"=w103, "Pop-up Config.Motor/VFD"=Motors_Type_Def."WB_Drag" ("Pop-up Config.Motor"), "Pop-up Config.Motor Type"=Motor_Type_Type_Def."MS", "Pop-up Config.Pop-up Corner"=Pop-up_Corner_Type_Def."Top Right") -> (w107:T20)
            n35 = Insert Into Array(array=w110, index=0, new element=string[] ["Update Motors", "Motor Pop-up"]) -> (w109:string[])
          }
          event Mouse Down {
            n36 = event-data() -> ("CtlRef"=w114:refnum<vi>)  [unwired: 1 in]
            n37 = Unbundle By Name(w113) -> ("Default Offset"=w112:T14)
            n38 = Bundle By Name(cluster=w113, "Pop-up Offset"=w112, "Selected Motor Ref"=w114, "Pop-up Config.Motor/VFD"=Motors_Type_Def."WS_Fan" ("Pop-up Config.Motor"), "Pop-up Config.Motor Type"=Motor_Type_Type_Def."MS", "Pop-up Config.Pop-up Corner"=Pop-up_Corner_Type_Def."Top Right") -> (w118:T20)
            n39 = Insert Into Array(array=w121, index=0, new element=string[] ["Update Motors", "Motor Pop-up"]) -> (w120:string[])
          }
          event Mouse Down {
            n40 = event-data() -> ("CtlRef"=w125:refnum<vi>)  [unwired: 1 in]
            n41 = Unbundle By Name(w124) -> ("Default Offset"=w123:T14)
            n42 = Bundle By Name(cluster=w124, "Pop-up Offset"=w123, "Selected Motor Ref"=w125, "Pop-up Config.Motor/VFD"=Motors_Type_Def."WB_Fan" ("Pop-up Config.Motor"), "Pop-up Config.Motor Type"=Motor_Type_Type_Def."MS", "Pop-up Config.Pop-up Corner"=Pop-up_Corner_Type_Def."Top Right") -> (w129:T20)
            n43 = Insert Into Array(array=w132, index=0, new element=string[] ["Update Motors", "Motor Pop-up"]) -> (w131:string[])
          }
          event Mouse Down {
            n44 = event-data() -> ("CtlRef"=w136:refnum<vi>)  [unwired: 1 in]
            n45 = Unbundle By Name(w135) -> ("Default Offset"=w134:T14)
            n46 = Bundle By Name(cluster=w135, "Pop-up Offset"=w134, "Selected Motor Ref"=w136, "Pop-up Config.Motor/VFD"=Motors_Type_Def."Dryer_Drag" ("Pop-up Config.Motor"), "Pop-up Config.Motor Type"=Motor_Type_Type_Def."MS", "Pop-up Config.Pop-up Corner"=Pop-up_Corner_Type_Def."Top Left") -> (w140:T20)
            n47 = Insert Into Array(array=w143, index=0, new element=string[] ["Update Motors", "Motor Pop-up"]) -> (w142:string[])
          }
          event Mouse Down {
            n48 = event-data() -> ("CtlRef"=w147:refnum<vi>)  [unwired: 1 in]
            n49 = Unbundle By Name(w146) -> ("Default Offset"=w145:T14)
            n50 = Bundle By Name(cluster=w146, "Pop-up Offset"=w145, "Selected Motor Ref"=w147, "Pop-up Config.Motor/VFD"=Motors_Type_Def."Dryer_Fan" ("Pop-up Config.Motor"), "Pop-up Config.Motor Type"=Motor_Type_Type_Def."MS", "Pop-up Config.Pop-up Corner"=Pop-up_Corner_Type_Def."Top Left") -> (w151:T20)
            n51 = Insert Into Array(array=w154, index=0, new element=string[] ["Update Motors", "Motor Pop-up"]) -> (w153:string[])
          }
          event Mouse Down {
            n52 = event-data() -> ("CtlRef"=w158:refnum<vi>)  [unwired: 1 in]
            n53 = Unbundle By Name(w157) -> ("Default Offset"=w156:T14)
            n54 = Bundle By Name(cluster=w157, "Pop-up Offset"=w156, "Selected Motor Ref"=w158, "Pop-up Config.Motor/VFD"=Motors_Type_Def."DB_Fan" ("Pop-up Config.Motor"), "Pop-up Config.Motor Type"=Motor_Type_Type_Def."VFD", "Pop-up Config.Pop-up Corner"=Pop-up_Corner_Type_Def."Bottom Left") -> (w162:T20)
            n55 = Insert Into Array(array=w165, index=0, new element=string[] ["Update Motors", "Motor Pop-up"]) -> (w164:string[])
          }
          event Mouse Down {
            n56 = event-data() -> ("CtlRef"=w171:refnum<vi>)  [unwired: 1 in]
            n57 = Unbundle By Name(w170) -> ("Default Offset"=w169:T14)
            n58 = Bundle By Name(cluster=w170, "Pop-up Offset"=w169, "Selected Motor Ref"=w171, "Pop-up Config.Motor/VFD"=Motors_Type_Def."DB_Drag" ("Pop-up Config.Motor"), "Pop-up Config.Motor Type"=Motor_Type_Type_Def."VFD", "Pop-up Config.Pop-up Corner"=Pop-up_Corner_Type_Def."Bottom Left", "Pop-up Offset.Top"=180, "Pop-up Offset.Left"=-10) -> (w175:T20)
            n59 = Insert Into Array(array=w178, index=0, new element=string[] ["Update Motors", "Motor Pop-up"]) -> (w177:string[])
          }
          event "DB_Top_Feed": Mouse Down {
            n60 = event-data() -> ("CtlRef"=w184:refnum<vi>)  [unwired: 1 in, 4 out]
            n61 = Unbundle By Name(w182) -> ("Default Offset"=w181:T14)
            n62 = Bundle By Name(cluster=w182, "Pop-up Offset"=w181, "Selected Motor Ref"=w184, "Pop-up Config.Motor/VFD"=Motors_Type_Def."DB_Top_Feed" ("Pop-up Config.Motor"), "Pop-up Config.Motor Type"=Motor_Type_Type_Def."VFD", "Pop-up Config.Pop-up Corner"=Pop-up_Corner_Type_Def."Bottom Left", "Pop-up Offset.Top"=325, "Pop-up Offset.Left"=3) -> (w188:T20)
            n63 = Insert Into Array(array=w191, index=0, new element=string[] ["Update Motors", "Motor Pop-up"]) -> (w190:string[])
          }
          event "Leg": Mouse Down {
            n64 = event-data() -> ("CtlRef"=w196:refnum<vi>)  [unwired: 1 in, 4 out]
            n65 = Bundle By Name(cluster=w197, "Selected Motor Ref"=w196, "Pop-up Config.Motor/VFD"=Motors_Type_Def."Leg" ("Pop-up Config.Motor"), "Pop-up Config.Motor Type"=Motor_Type_Type_Def."VFD", "Pop-up Config.Pop-up Corner"=Pop-up_Corner_Type_Def."Top Left", "Pop-up Offset.Left"=-125, "Pop-up Offset.Top"=-210) -> (w200:T20)
            n66 = Insert Into Array(array=w203, index=0, new element=string[] ["Update Motors", "Motor Pop-up"]) -> (w202:string[])
          }
          event "Motor_Toggle": Value Change {
            n67 = event-data() -> ()  [unwired: 1 in, 6 out]
            n68 = Bundle By Name(cluster=w206, "Motor Toggle"="Motor_Toggle") -> (w205:T20)
            n69 = Insert Into Array(array=w210, index=0, new element=string[] ["Motor/VFD Toggle"]) -> (w209:string[])
          }
          event "VFD_Toggle": Value Change {
            n70 = event-data() -> ()  [unwired: 1 in, 6 out]
            n71 = Bundle By Name(cluster=w213, "Motor Toggle"="VFD_Toggle") -> (w212:T20)
            n72 = Insert Into Array(array=w217, index=0, new element=string[] ["Motor/VFD Toggle"]) -> (w216:string[])
          }
          event "VFD_+1", "VFD_+0.1", "VFD_-0.1", "VFD_-1": Value Change {
            n73 = event-data() -> ()  [unwired: 1 in, 6 out]
            n74 = Unbundle By Name(w223) -> ("VFD_CMD"=w222:dbl)
            n75 = Build Array("VFD_+1", "VFD_+0.1", "VFD_-0.1", "VFD_-1") -> (w226:bool[])
            n76 = call "Search Unsorted 1D Array.vim"("element"=TRUE, "unsorted 1D array"=w226) -> ("index of element"=w224:i32)  [unwired: 9 in]
            n77 = case shown="3" w224 {
              tunnel: w222 -> [w237 w240 w243 w244]
              tunnel: [w236 w238 w241 w245] -> w221
              frame 0, Default {
                n78 = Increment(x=w237) -> (x+1=w236:dbl)
              }
              frame 1 {
                n79 = Add(x=w240, y=0.1) -> (x+y=w238:dbl)
              }
              frame 2 {
                n80 = Subtract(x=w243, y=0.1) -> (x-y=w241:dbl)
              }
              frame 3 {
                n81 = Decrement(x=w244) -> (x-1=w245:dbl)
              }
            }
            n82 = In Range and Coerce(upper limit=60.0, x=w221, lower limit=0.0) -> (coerced(x)=w220:dbl)  [unwired: 1 out]
            n83 = Bundle By Name(cluster=w223, "VFD_CMD"=w220) -> (w231:T20)
            n84 = Insert Into Array(array=w235, index=0, new element=string[] ["Send VFD CMD"]) -> (w234:string[])
          }
          event "VFD_CMD": Value Change {
            n85 = event-data() -> ()  [unwired: 1 in, 6 out]
            n86 = Bundle By Name(cluster=w247, "VFD_CMD"="VFD_CMD") -> (w248:T20)
            n87 = Insert Into Array(array=w252, index=0, new element=string[] ["Send VFD CMD"]) -> (w251:string[])
          }
          event "VFD_CMD": Mouse Down {
            n88 = event-data() -> ()  [unwired: 1 in, 8 out]
            n89 = property on="Settings Pop-up" class="TabCtl (strict)"("Position"=T14 {"Left"=-1073, "Top"=-150}) -> ()  [unwired: 2 in, 2 out]
            n90 = constructor class="Process"() -> (reference out=w255:refnum<k24>)  [unwired: 3 in, 2 out]
            n91 = invoke class="Process" method="Start"(reference=w255, "fileName"="C:\\Program Files\\Common Files\\Microsoft Shared\\Ink\\TabTip.exe") -> ()  [unwired: 2 in, 4 out]
            n92 = Insert Into Array(array=w260, index=0, new element=string[] []) -> (w259:string[])
          }
          event "Shutdown": Value Change {
            n93 = event-data() -> ()  [unwired: 1 in, 6 out]
            n94 = Bundle By Name(cluster=w264, "Info Config.Title"="ATTENTION", "Info Config.Message"="This will stop Auto Mode, and turn off all augers and drags.", "Info Config.Next State"="Shutdown") -> (w265:T20)
            n95 = Insert Into Array(array=w269, index=0, new element=string[] ["Info Pop-up"]) -> (w268:string[])
          }
          event "Auto/Manual PB": Value Change {
            n96 = event-data() -> ()  [unwired: 1 in, 6 out]
            n97 = Bundle By Name(cluster=w271, "Mode Toggle"="Auto/Manual PB") -> (w272:T20)
            n98 = Insert Into Array(array=w276, index=0, new element=string[] ["Mode Toggle"]) -> (w275:string[])
          }
          event "Info Ok PB": Value Change {
            n99 = event-data() -> ()  [unwired: 1 in, 6 out]
            n100 = Unbundle By Name(w282) -> ("Info Config.Next State"=w278:string)
            n101 = Build Array(w278) -> (w277:string[])
            n102 = Insert Into Array(array=w280, index=0, new element=w277) -> (w279:string[])
            n103 = Insert Into Array(array=w279, index=0, new element=string[] ["Hide Pop-ups"]) -> (w285:string[])
          }
          event "Info Cancel PB": Value Change {
            n104 = event-data() -> ()  [unwired: 1 in, 6 out]
            n105 = Insert Into Array(array=w286, index=0, new element=string[] ["Hide Pop-ups"]) -> (w290:string[])
          }
          event "Alarm Ok PB": Value Change {
            n106 = event-data() -> ()  [unwired: 1 in, 6 out]
            n107 = Insert Into Array(array=w295, index=0, new element=string[] ["Hide Pop-ups"]) -> (w294:string[])
          }
          event "Settings PB": Value Change {
            n108 = event-data() -> ()  [unwired: 1 in, 6 out]
            n109 = Insert Into Array(array=w300, index=0, new element=string[] ["Settings Pop-up"]) -> (w299:string[])
          }
          event "Settings Ok PB": Value Change {
            w304 = 0  # Leg Dry Limit
            n110 = event-data() -> ()  [unwired: 1 in, 6 out]
            n111 = Unbundle By Name(w310) -> ("Email Config Path"=w312:path)
            n112 = Write to Binary File(file (use dialog)=w312, data="Email Config") -> ()  [unwired: 4 in, 3 out]
            n113 = Unbundle By Name("Auto Params 2") -> ("Top Fd Auto Spd:"=w316:dbl)
            n114 = Cluster To Array(cluster="Auto Params 1") -> (array=w306:T6[])
            n115 = Cluster To Array(cluster="Alarm Limits") -> (array=w307:T6[])
            n116 = Delete From Array(array=w306, length=1, index=w304) -> (deleted portion=w302:T6[], array with subset deleted=w303:T6[])
            n117 = Index Array(array=w302) -> (element=w301:T6)  [unwired: 1 in]
            n118 = Multiply(x=w316, y=100.0) -> (x*y=w314:dbl)
            n119 = To Unsigned Word Integer(number=w314) -> (unsigned 16bit integer=w313:u16)
            n120 = Build Array (concatenate)(w303, w313, w307, w301) -> (w318:T6[])
            n121 = call "Modbus Global.vi"("Modbus Mode (Write Coil)"=Modbus_Mode."Param Write", "Params IN"=w318) -> ()  [unwired: 10 in, 4 out]
            n122 = Bundle By Name(cluster=w310, "Email Config"="Email Config") -> (w311:T20)
            n123 = Insert Into Array(array=w324, index=0, new element=string[] ["Hide Pop-ups"]) -> (w323:string[])
          }
          event "Settings Cancel PB": Value Change {
            n124 = event-data() -> ()  [unwired: 1 in, 6 out]
            n125 = Insert Into Array(array=w329, index=0, new element=string[] ["Hide Pop-ups"]) -> (w328:string[])
          }
          event "Reset Leg Dry PB": Value Change {
            n126 = event-data() -> ()  [unwired: 1 in, 6 out]
            n127 = call "Modbus Global.vi"("HMI Coil"=HMI_Coils."MC122_HMI_Reset_Leg_Dry", "Modbus Mode (Write Coil)"=Modbus_Mode."Write Coil", "Coil IN"=TRUE) -> ()  [unwired: 9 in, 4 out]
            n128 = Insert Into Array(array=w337, index=0, new element=string[] []) -> (w336:string[])
          }
          event "Exit": Mouse Down {
            n129 = event-data() -> ("Mods"=w339:cluster{"Double Click":bool, "Menu Key":bool})  [unwired: 1 in, 7 out]
            n130 = Unbundle By Name(w339) -> ("Double Click"=w338:bool)
            n131 = case shown="True" w338 {
              tunnel: [string[] [] string[] ["Exit"]] -> w341
              frame False {
              }
              frame True {
              }
            }
            n132 = Insert Into Array(array=w344, index=0, new element=w341) -> (w343:string[])
          }
        }
      }
      frame "Init" {
        n133 = local write "Exit"(FALSE ("Exit")) -> ()
        n134 = Insert Into Array(array=w350, index=0, new element=string[] []) -> (w349:string[])
      }
      frame "Init Alarms" {
        n135 = Array Size(array="Alarms") -> (size(s)=w354:i32)
        n136 = Initialize Array(FALSE, w354) -> (w353:bool[])
        n137 = Bundle By Name(cluster=w357, "Alarms"="Alarms", "Prev Alarm States"=w353) -> (w358:T20)
        n138 = Insert Into Array(array=w360, index=0, new element=string[] []) -> (w359:string[])
      }
      frame "Init Refs" {
        n139 = control-ref of="WS_Drag"() -> (w377:refnum<vi>)
        n140 = control-ref of="WB_Drag"() -> (w376:refnum<vi>)
        n141 = control-ref of="WS_Fan"() -> (w375:refnum<vi>)
        n142 = control-ref of="WB_Fan"() -> (w374:refnum<vi>)
        n143 = control-ref of="Dryer_Drag"() -> (w373:refnum<vi>)
        n144 = control-ref of="Dryer_Fan"() -> (w372:refnum<vi>)
        n145 = control-ref of="DB_Fan"() -> (w371:refnum<vi>)
        n146 = control-ref of="DB_Drag"() -> (w370:refnum<vi>)
        n147 = control-ref of="DB_Top_Feed"() -> (w369:refnum<vi>)
        n148 = control-ref of="U-Trough"() -> (w363:refnum<vi>)
        n149 = control-ref of="Leg"() -> (w368:refnum<vi>)
        n150 = Build Array(w377, w376, w375, w374, w373, w372, w371, w370, w369, w363, w368) -> (w367:refnum<vi>[])
        n151 = Array Size(array=w367) -> (size(s)=w366:i32)
        n152 = for {
          tunnel: w367 -> [w384] mode=indexing
          n153 = property class="Bool (strict)"(reference=w384, "Value"=FALSE) -> ()  [unwired: 1 in, 2 out]
        }
        n154 = Initialize Array(T23 {"Running"=FALSE, "OL/Fault"=FALSE, "VFD Speed"=0.0, "VFD CMD"=0.0} ("Motor Data"), w366) -> (w364:T28)
        n155 = Bundle By Name(cluster=w378, "Motor Refs"=w367, "Motor Data"=w364) -> (w379:T20)
        n156 = Insert Into Array(array=w381, index=0, new element=string[] []) -> (w380:string[])
      }
      frame "Init Bins" {
        n157 = control-ref of="DB_Scale"() -> (w403:refnum<vi>)
        n158 = control-ref of="DB_Background"() -> (w404:refnum<vi>)
        n159 = control-ref of="WB_Scale"() -> (w406:refnum<vi>)
        n160 = control-ref of="WB_Background"() -> (w407:refnum<vi>)
        n161 = control-ref of="WS_Scale"() -> (w411:refnum<vi>)
        n162 = control-ref of="WS_Background"() -> (w410:refnum<vi>)
        n163 = control-ref of="Dryer_Scale"() -> (w393:refnum<vi>)
        n164 = control-ref of="Dryer_Background"() -> (w392:refnum<vi>)
        n165 = control-ref of="DB_Numeric"() -> (w405:refnum<vi>)
        n166 = control-ref of="WB_Numeric"() -> (w408:refnum<vi>)
        n167 = control-ref of="WS_Numeric"() -> (w409:refnum<vi>)
        n168 = control-ref of="Dryer_Numeric"() -> (w391:refnum<vi>)
        n169 = Bundle By Name(cluster=T24 {"Scale"=refnum, "Background"=refnum, "Numeric"=refnum, "Bin Max"=0} ("Bin Indicator Refs"), "Scale"=w403, "Background"=w404, "Numeric"=w405, "Bin Max"=u16 49373) -> (w395:T24)
        n170 = Bundle By Name(cluster=T24 {"Scale"=refnum, "Background"=refnum, "Numeric"=refnum, "Bin Max"=0} ("Bin Indicator Refs"), "Scale"=w406, "Background"=w407, "Numeric"=w408, "Bin Max"=u16 11025) -> (w387:T24)
        n171 = Bundle By Name(cluster=T24 {"Scale"=refnum, "Background"=refnum, "Numeric"=refnum, "Bin Max"=0} ("Bin Indicator Refs"), "Scale"=w411, "Background"=w410, "Numeric"=w409, "Bin Max"=u16 8865) -> (w388:T24)
        n172 = Bundle By Name(cluster=T24 {"Scale"=refnum, "Background"=refnum, "Numeric"=refnum, "Bin Max"=0} ("Bin Indicator Refs"), "Scale"=w393, "Background"=w392, "Numeric"=w391, "Bin Max"=u16 4128) -> (w386:T24)
        n173 = Build Array(w395, w386, w387, w388) -> (w394:T24[])
        n174 = call "Bin Indicator Control.vi"("Bin Indicator Refs"=w394, "Init (F)"=TRUE) -> ()  [unwired: 14 in]
        n175 = Insert Into Array(array=w414, index=0, new element=string[] []) -> (w413:string[])
      }
      frame "Get Email Config" {
        n176 = Unbundle By Name(w420) -> ("Email Config"=w422:T9[])
        n177 = call <vilib>:"Application Directory.vi"() -> ("Application Directory"=w424:path)
        n178 = Build Path(base path=w424, name or relative path=path "Email Config") -> (appended path=w417:path)
        n179 = Read from Binary File(5:w422, 11:w417) -> (0:w418:errorcluster, 2:w419:T9[])  [unwired: 4 in, 2 out]
        n180 = call <vilib>:"Clear Errors.vi"("error in (no error)"=w418) -> ()  [unwired: 5 in, 2 out]
        n181 = Bundle By Name(cluster=w420, "Email Config Path"=w417, "Email Config"=w419) -> (w421:T20)
        n182 = Insert Into Array(array=w426, index=0, new element=string[] []) -> (w425:string[])
      }
      frame "Unused Items" {
        n183 = Insert Into Array(array=w431, index=0, new element=string[] []) -> (w430:string[])
      }
      frame "Check Connection" {
        n184 = Unbundle By Name(w442) -> ("Heartbeat Timer"=w448:u32, "Connected"=w445:bool)
        n185 = Tick Count (ms)() -> (millisecond timer value=w446:u32)
        n186 = Subtract(x=w446, y=w448) -> (x-y=w450:u32)
        n187 = Greater?(x=w450, y=u32 200) -> (0:w449:bool)
        n188 = case shown="False" w449 {
          tunnel: [w467 w469] -> w447
          tunnel: w448 -> [w467 _]
          tunnel: w446 -> [_ w469]
          tunnel: [w466 w470] -> w438
          tunnel: w445 -> [w466 _]
          frame False {
          }
          frame True {
            n189 = local read "Heartbeat OUT"() -> (w468:bool)
            "Heartbeat IN" <- w468
            n190 = feedback #1() -> (w471:bool)  [unwired: 1 in]
            n191 = feedback-in #1(w468) -> ()
            n192 = Not Equal?(x=w468, y=w471) -> (x != y?=w470:bool)
          }
        }
        n193 = feedback #2() -> (w440:bool)  [unwired: 1 in]
        n194 = feedback-in #2(w438) -> ()
        n195 = case shown="True" w438 {
          tunnel: [string[] [] string[] ["Update Motors", "Update Screen", "Check Alarms"]] -> w441
          frame False {
          }
          frame True {
          }
        }
        n196 = Not Equal?(x=w438, y=w440) -> (x != y?=w439:bool)
        n197 = case shown="True" w439 {
          tunnel: w438 -> [_ w458]
          tunnel: [string[] [] w456] -> w434
          frame False {
          }
          frame True {
            n198 = case shown="False" w458 {
              tunnel: [TRUE ("Visible") FALSE ("Visible")] -> w459
              tunnel: [T25."Disabled and Grayed Out" ("Disabled") T25."Enabled" ("Disabled")] -> w457
              tunnel: [string[] ["Hide Pop-ups"] string[] []] -> w456
              frame False {
              }
              frame True {
              }
            }
            n199 = property on="PLC Disconnected" class="Str"("Visible"=w459) -> ()  [unwired: 2 in, 2 out]
            n200 = property on="Main Tab" class="TabCtl (strict)"("DisabledEnum"=w457) -> ()  [unwired: 2 in, 2 out]
          }
        }
        n201 = Insert Into Array(array=w451, index=0, new element=w441) -> (w436:string[])
        n202 = Bundle By Name(cluster=w442, "Heartbeat Timer"=w447, "Connected"=w438) -> (w443:T20)
        n203 = Insert Into Array(array=w436, index=0, new element=w434) -> (w435:string[])
      }
      frame "Update Motors" {
        w472 = 8  # Top Feed
        w473 = 10  # Leg
        n204 = Unbundle By Name(w480) -> ("Pop-up Config.Motor Type"=w489:T17, "Pop-up Config.Motor/VFD"=w486:T16, "Motor Refs"=w490:refnum<vi>[], "PLC Coils"=w488:bool[], "PLC Regs"=w487:u16[], "Motor Data"=w479:T13[])
        n205 = call "Update Motors.vi"("VFD Refs"=w490, "PLC Coils"=w488, "PLC Regs"=w487, "Motor Data IN"=w479) -> ("Motor Data OUT"=w477:T28)  [unwired: 15 in]
        n206 = Index Array(array=w477, index=w486) -> (element=w485:T23)
        n207 = Index Array(array=w477, index #1=w472, index #2=w473) -> (element #1=w478:T23, element #2=w474:T23)
        n208 = Unbundle By Name(w485) -> ("Running"=w484:bool, "OL/Fault"=w483:bool, "VFD Speed"=w482:dbl)
        n209 = Unbundle By Name(w478) -> ("Running"=w476:bool)
        n210 = Unbundle By Name(w474) -> ("Running"=w475:bool)
        n211 = case shown="\"VFD\"" w489 {
          tunnel: w484 -> [w496 w499]
          tunnel: w483 -> [w495 w498]
          tunnel: w482 -> [_ w497]
          frame "MS", Default {
            "Motor_Running" <- w496
            "Motor_Overload" <- w495
          }
          frame "VFD" {
            "VFD_Running" <- w499
            "VFD_Fault" <- w498
            "VFD_Speed" <- w497
          }
        }
        n212 = property on="DB Tp Fd Amps" class="DigNum (strict)"("Visible"=w476) -> ()  [unwired: 2 in, 2 out]
        n213 = property on="Leg_Amps" class="DigNum (strict)"("Visible"=w475) -> ()  [unwired: 2 in, 2 out]
        n214 = Bundle By Name(cluster=w480, "Motor Data"=w477) -> (w481:T20)
        n215 = Insert Into Array(array=w492, index=0, new element=string[] []) -> (w491:string[])
      }
      frame "Update Screen" {
        w507 = 100.0 ("y")
        w526 = T26[] [enum."MHR220_PLC_DB_Level", enum."MHR223_PLC_Dryr_Bin_Level", enum."MHR221_PLC_WB_Level", enum."MHR222_PLC_WS_Level"] items=["MHR200_PLC_DB_Fan_Spd", "MHR201_PLC_DB_Drag_Spd", "MHR202_PLC_DB_Tp_Fd_Spd", "MHR203_PLC_U_Trough_Spd", "MHR204_PLC_Leg_Spd", "MHR205_PLC_DB_Fan_ON", "MHR206_PLC_DB_Drag_ON", "MHR207_PLC_DB_Tp_Fd_ON", "MHR208_PLC_U_Trough_ON", "MHR209_PLC_Leg_ON", "MHR210_PLC_DB_Fan_CMD", "MHR211_PLC_DB_Drag_CMD", "MHR212_PLC_DB_Tp_Fd_CMD", "MHR213_PLC_U_Trough_CMD", "MHR214_PLC_Leg_CMD", "MHR215_PLC_DB_Fan_Flt", "MHR216_PLC_DB_Drag_Flt", "MHR217_PLC_DB_Tp_Fd_Flt", "MHR218_PLC_U_Trough_Flt", "MHR219_PLC_Leg_Flt", "MHR220_PLC_DB_Level", "MHR221_PLC_WB_Level", "MHR222_PLC_WS_Level", "MHR223_PLC_Dryr_Bin_Level", "MHR224_PLC_Leg_Amps", "MHR225_PLC_DB_Tp_Fd_Amps"]
        w531 = T2[] [enum."MC200_PLC_Estop_Main", enum."MC201_PLC_Estop_GSI", enum."MC202_PLC_Estop_Dryer", enum."MC260_PLC_Dryer_Full", enum."MC261_PLC_Dryer_HI_Alm", enum."MC262_PLC_Dryr_Bin_Full", enum."MC263_PLC_DB_HI_Alm", enum."MC265_PLC_Dryer_Feed", enum."MC203_PLC_Auto_Mode", enum."MC270_PLC_WS_Limit", enum."MC271_PLC_WB_Limit", enum."MC272_PLC_Dryr_Bin_Lim", enum."MC273_PLC_DB_Limit", enum."MC264_PLC_Dryer_Chute", enum."MC274_PLC_Auto_Leg_Dry"] items=["MC200_PLC_Estop_Main", "MC201_PLC_Estop_GSI", "MC202_PLC_Estop_Dryer", "MC203_PLC_Auto_Mode", "MC204", "MC205", "MC206", "MC207", "MC208", "MC209", "MC210", "MC211", "MC212", "MC213", "MC214", "MC215", "MC216", "MC217", "MC218", "MC219", "MC220_PLC_WS_Drag_ON", "MC221_PLC_WB_Drag_ON", "MC222_PLC_WS_Fan_ON", "MC223_PLC_WB_Fan_ON", "MC224_PLC_Dryr_Drag_ON", "MC225_PLC_Dryr_Fan_ON", "MC226", "MC227", "MC228", "MC229", "MC230", "MC231", "MC232", "MC233", "MC234", "MC235", "MC236", "MC237", "MC238", "MC239", "MC240_PLC_WS_Drag_OL", "MC241_PLC_WB_Drag_OL", "MC242_PLC_WS_Fan_OL", "MC243_PLC_WB_Fan_OL", "MC244_PLC_Dryr_Drag_OL", "MC245_PLC_Dryr_Fan_OL", "MC246_PLC_DB_Fan_Alm", "MC247_PLC_DB_Drag_Alm", "MC248_PLC_DB_Tp_Fd_Alm", "MC249_PLC_U_Trough_Alm", "MC250_PLC_Leg_Alm", "MC251", "MC252", "MC253", "MC254", "MC255", "MC256", "MC257", "MC258", "MC259", "MC260_PLC_Dryer_Full", "MC261_PLC_Dryer_HI_Alm", "MC262_PLC_Dryr_Bin_Full", "MC263_PLC_DB_HI_Alm", "MC264_PLC_Dryer_Chute", "MC265_PLC_Dryer_Feed", "MC266", "MC267", "MC268", "MC269", "MC270_PLC_WS_Limit", "MC271_PLC_WB_Limit", "MC272_PLC_Dryr_Bin_Lim", "MC273_PLC_DB_Limit", "MC274_PLC_Auto_Leg_Dry", "MC275", "MC276", "MC277", "MC278", "MC279", "MC280_Auto_Error_0", "MC281_Auto_Error_1", "MC282_Auto_Error_2", "MC283_Auto_Error_3", "MC284_Auto_Error_4", "MC285_Auto_Error_5", "MC286_Auto_Error_6", "MC287_Auto_Error_7", "MC288_Auto_Error_8", "MC289_Auto_Error_9"]
        n216 = Unbundle By Name(w533) -> ("PLC Coils"=w532:bool[], "PLC Regs"=w515:u16[], "debug"=w503:bool)
        n217 = for {
          tunnel: w532 -> [w543]
          tunnel: w531 -> [w542] mode=indexing
          tunnel: [w541] -> w530 mode=indexing
          n218 = Index Array(array=w543, index=w542) -> (element=w541:bool)
        }
        n219 = for {
          tunnel: w515 -> [w540]
          tunnel: w526 -> [w539] mode=indexing
          tunnel: [w538] -> w502 mode=indexing
          n220 = Index Array(array=w540, index=w539) -> (element=w538:u16)
        }
        n221 = Index Array(array=w515, index #1=PLC_Registers."MHR224_PLC_Leg_Amps" ("PLC Reg"), index #2=PLC_Registers."MHR225_PLC_DB_Tp_Fd_Amps" ("PLC Reg")) -> (element #1=w513:u16, element #2=w506:u16)
        n222 = To Double Precision Float(number=w513) -> (double precision float=w512:dbl)
        n223 = To Double Precision Float(number=w506) -> (double precision float=w508:dbl)
        n224 = Select(t="Array", s=w503, f=w502) -> (s? t:f=w501:u16[])
        "Bin Levels" <- w501
        n225 = Index Array(array=w530) -> (element #1=→"E-Stop (Main)":bool, element #2=→"E-Stop (GSI)":bool, element #3=→"E-Stop (Dryer)":bool, element #4=→"Dryer Full":bool, element #5=→"Dryer High Alarm":bool, element #6=→"Dryer Bin Full":bool, element #7=→"Dry Bin High Alarm":bool, element #8=→"Dryer Feed":bool, element #9=→"Auto Mode":bool, element #10=→"Wet Silo Level Limit":bool, element #11=→"Wet Bin Level Limit":bool, element #12=→"Dryer Bin Level Limit":bool, element #13=→"Dry Bin Level Limit":bool, element #14=→"Dryer Chute Open":bool, element #15=w504:bool)  [unwired: 15 in]
        "Leg Dry Run" <- w504
        n226 = Divide(x=w512, y=w507) -> (x/y=→"Leg_Amps":dbl)
        n227 = Divide(x=w508, y=w507) -> (x/y=→"DB Tp Fd Amps":dbl)
        n228 = call "Bin Indicator Control.vi"("Bin Levels"=w501) -> ()  [unwired: 15 in]
        n229 = property on="Leg Dry Run" class="Bool (strict)"("Visible"=w504) -> ()  [unwired: 2 in, 2 out]
        n230 = property on="Reset Leg Dry PB" class="Bool (strict)"("Visible"=w504) -> ()  [unwired: 2 in, 2 out]
        n231 = Insert Into Array(array=w535, index=0, new element=string[] []) -> (w534:string[])
      }
      frame "Check Alarms" {
        n232 = Unbundle By Name(w556) -> ("PLC Coils"=w547:bool[], "Prev Alarm States"=w548:bool[], "Alarms"=w553:T1[], "Active Alarm Config"=w546:T1, "Active Alarm"=w550:bool, "Active Alarm Config.Alarm Type"=w552:T3)
        n233 = Equal?(x=w552, y=Alarm_Type."Emergency") -> (x = y?=w549:bool)
        n234 = for {
          tunnel: w547 -> [w576]
          tunnel: w553 -> [w575] mode=indexing
          tunnel: [w573] -> w544 mode=indexing
          n235 = Unbundle By Name(w575) -> ("PLC Coil"=w574:T2)
          n236 = Index Array(array=w576, index=w574) -> (element=w573:bool)
        }
        n237 = And(x=w550, y=w549) -> (x .and. y?=w545:bool)
        n238 = case shown="False" w545 {
          tunnel: [w566 w572] -> w555
          tunnel: [w565 FALSE] -> w554
          tunnel: w553 -> [w564 _]
          tunnel: w548 -> [w563 _]
          tunnel: w544 -> [w562 _]
          tunnel: w546 -> [_ w572]
          frame False {
            # "Check alarms if there isn't\nan active Emergency."
            n239 = for {
              tunnel: w564 -> [w567] mode=indexing
              tunnel: [w570] -> w565
              tunnel: [w567] -> w566
              tunnel: w563 -> [w569] mode=indexing
              tunnel: w562 -> [w568] mode=indexing
              stop <- w570 stop-if-true
              n240 = Greater?(x=w568, y=w569) -> (0:w570:bool)
            }
          }
          frame True {
          }
        }
        n241 = case shown="True" w554 {
          tunnel: [string[] [] string[] ["Handle Alarm"]] -> w560
          frame False {
          }
          frame True {
          }
        }
        n242 = Bundle By Name(cluster=w556, "Prev Alarm States"=w544, "Active Alarm Config"=w555) -> (w557:T20)
        n243 = Insert Into Array(array=w559, index=0, new element=w560) -> (w558:string[])
      }
      frame "Handle Alarm" {
        n244 = Unbundle By Name(w597) -> ("Active Alarm Config.Message"=→"Alarm Message":string, "Active Alarm Config.Alarm Type"=w591:T3, "Active Alarm Config.Shutdown"=w587:bool, "Active Alarm Config.Send Email"=w582:bool)
        n245 = case shown="\"Emergency\"" w591 {
          tunnel: [u32 0 u32 16777215] -> w594
          tunnel: [u32 16775210 u32 16711680] -> w593
          tunnel: ["WARNING" ("Alarm Title") "EMERGENCY!" ("Alarm Title")] -> w592
          frame "Warning", Default {
          }
          frame "Emergency" {
          }
        }
        n246 = case shown="True" w582 {
          tunnel: [string[] [] string[] ["Alarm Email"]] -> w586
          frame False {
          }
          frame True {
          }
        }
        n247 = property on="Alarm Title" class="Str"("Text.TextColor"=w594, "Text.BGColor"=w593, "Value"=w592) -> (error out=w581:errorcluster)  [unwired: 2 in, 1 out]
        n248 = call "Stall Data Flow.vim"("value in"=w581, "milliseconds to wait"=u32 50) -> ("value out"=w580:errorcluster)  [unwired: 1 out]
        n249 = Insert Into Array(array=w584, index=0, new element=w586) -> (w583:string[])
        n250 = property on="Alarm Pop-up" class="TabCtl (strict)"(error in=w580, "Visible"=TRUE) -> (error out=w588:errorcluster)  [unwired: 1 in, 1 out]
        n251 = case shown="True" w587 {
          tunnel: [string[] [] string[] ["Shutdown"]] -> w600
          frame False {
          }
          frame True {
          }
        }
        n252 = property on="Main Tab" class="TabCtl (strict)"(error in=w588, "DisabledEnum"=T25."Disabled and Grayed Out" ("Disabled")) -> ()  [unwired: 1 in, 2 out]
        n253 = Bundle By Name(cluster=w597, "Active Alarm"=TRUE) -> (w598:T20)
        n254 = Insert Into Array(array=w583, index=0, new element=w600) -> (w599:string[])
      }
      frame "Alarm Email" {
        n255 = Unbundle By Name(w615) -> ("Active Alarm Config.Message"=w613:string, "Email Config"=w612:T9[])
        n256 = call "Email Global.vi"("Write (F)"=TRUE, "Emails IN"=w612, "Message IN"=w613) -> ()  [unwired: 6 in, 3 out]
        n257 = Insert Into Array(array=w617, index=0, new element=string[] []) -> (w616:string[])
      }
      frame "Info Pop-up" {
        n258 = Unbundle By Name(w620) -> ("Info Config.Title"=w622:string, "Info Config.Message"=w621:string)
        n259 = flat-sequence {
          tunnel: w622 -> [w628]
          tunnel: w621 -> [w627]
          frame #0 {
            "Info Title" <- w628
            "Info Message" <- w627
          }
          frame #1 {
            n260 = Wait (ms)(milliseconds to wait=u32 50) -> ()  [unwired: 1 out]
          }
          frame #2 {
            n261 = property on="Info Pop-up" class="TabCtl (strict)"("Visible"=TRUE) -> (error out=w632:errorcluster)  [unwired: 2 in, 1 out]
            n262 = property on="Main Tab" class="TabCtl (strict)"(error in=w632, "DisabledEnum"=T25."Disabled and Grayed Out" ("Disabled")) -> ()  [unwired: 1 in, 2 out]
          }
        }
        n263 = Insert Into Array(array=w624, index=0, new element=string[] []) -> (w623:string[])
      }
      frame "Settings Pop-up" {
        n264 = flat-sequence {
          tunnel: w633 -> [w642]
          frame #0 {
            n265 = Unbundle By Name(w642) -> ("debug"=w640:bool, "Email Config"=w641:T9[])
            n266 = case shown="False" w640 {
              frame False {
                n267 = call "Modbus Global.vi"("Modbus Mode (Write Coil)"=Modbus_Mode."Param Read") -> ("Params OUT"=w645:u16[])  [unwired: 11 in, 3 out]
                n268 = Index Array(array=w645, index=10) -> (element=w644:u16)
                n269 = Array Subset(array=w645, index=0, length=5) -> (w647:u16[])
                n270 = Index Array(array=w645, index=5) -> (element=w652:u16)
                n271 = Array Subset(array=w645, index=6, length=4) -> (w649:u16[])
                n272 = To Double Precision Float(number=w652) -> (double precision float=w655:dbl)
                n273 = Build Array (concatenate)(w644, w647) -> (w643:u16[])
                n274 = Divide(x=w655, y=100.0) -> (x/y=w654:dbl)
                n275 = Bundle(w654) -> (w653:cluster{dbl})  [unwired: 1 in]
                n276 = Array To Cluster(array=w643) -> (cluster=w658:T29)
                n277 = Array To Cluster(array=w649) -> (cluster=w648:T30)
                n278 = local write "Auto Params 1"(w658) -> ()
                n279 = local write "Auto Params 2"(w653) -> ()
                n280 = local write "Alarm Limits"(w648) -> ()
              }
              frame True {
              }
            }
            n281 = local write "Email Config"(w641) -> ()
          }
          frame #1 {
            n282 = Wait (ms)(milliseconds to wait=u32 100) -> ()  [unwired: 1 out]
          }
          frame #2 {
            n283 = property on="Settings Pop-up" class="TabCtl (strict)"("Position"=T14 {"Left"=-890, "Top"=-150}, "Visible"=TRUE) -> (error out=w666:errorcluster)  [unwired: 2 in, 1 out]
            n284 = property on="Settings Tab" class="TabCtl (strict)"(error in=w666, "Value"=T4."Auto Params" ("Settings Tab")) -> (error out=w665:errorcluster)  [unwired: 1 in, 1 out]
            n285 = property on="Main Tab" class="TabCtl (strict)"(error in=w665, "DisabledEnum"=T25."Disabled and Grayed Out" ("Disabled")) -> ()  [unwired: 1 in, 2 out]
          }
        }
        n286 = Bundle By Name(cluster=w633, "Params Open"=TRUE) -> (w635:T20)
        n287 = Insert Into Array(array=w637, index=0, new element=string[] []) -> (w636:string[])
      }
      frame "Motor Pop-up" {
        n288 = Unbundle By Name(w672) -> ("Motor Data"=w671:T13[], "Pop-up Config.Motor/VFD"=w670:T16, "Pop-up Config"=w678:T15, "Pop-up Offset"=w677:T14, "Selected Motor Ref"=w676:refnum<vi>, "Motor Descriptions"=w675:string[])
        n289 = Index Array(array=w671, index=w670) -> (element=w674:T13)
        n290 = Unbundle By Name(w674) -> ("VFD CMD"=w669:dbl)
        n291 = local write "VFD_CMD"(w669) -> ()
        n292 = flat-sequence {
          tunnel: w678 -> [w691]
          tunnel: w677 -> [w690]
          tunnel: w676 -> [w689]
          tunnel: w675 -> [w688]
          tunnel: w669 -> [_]
          frame #0 {
            n293 = control-ref of="Main Tab"() -> (w687:refnum<vi>)
            n294 = control-ref of="Motor Pop-up"() -> (w693:refnum<vi>)
            n295 = control-ref of="VFD Pop-up"() -> (w692:refnum<vi>)
            n296 = control-ref of="Motor_Sel (Round)"() -> (w686:refnum<vi>)
            n297 = control-ref of="Motor_Sel (Square)"() -> (w685:refnum<vi>)
            n298 = control-ref of="Motor_Title"() -> (w684:refnum<vi>)
            n299 = control-ref of="VFD_Title"() -> (w683:refnum<vi>)
            n300 = call "Pop-up Config.vi"("Motor Pop-up Config"=w691, "Offset"=w690, "Motor Indicator"=w689, "Motor Pop-up"=w693, "VFD Pop-up"=w692, "Motor_Title"=w684, "Main Tab"=w687, "VFD_Title"=w683, "Motor Descriptions"=w688, "Motor_Sel (Round)"=w686, "Motor_Sel (Square)"=w685) -> ()  [unwired: 9 in]
          }
        }
        n301 = Bundle By Name(cluster=w672, "VFD_CMD"=w669) -> (w673:T20)
        n302 = Insert Into Array(array=w680, index=0, new element=string[] []) -> (w679:string[])
      }
      frame "Hide Pop-ups" {
        w701 = FALSE ("Active Alarm")
        w702 = FALSE ("Visible")
        n303 = Unbundle By Name(w700) -> ("Connected"=w696:bool, "debug"=w695:bool)
        n304 = Or(x=w696, y=w695) -> (x .or. y?=w694:bool)
        n305 = Select(t=T25."Enabled" ("Disabled"), s=w694, f=T25."Disabled and Grayed Out" ("Disabled")) -> (s? t:f=w698:T25)
        n306 = property on="Motor Pop-up" class="TabCtl (strict)"("Visible"=w702) -> ()  [unwired: 2 in, 2 out]
        n307 = property on="VFD Pop-up" class="TabCtl (strict)"("Visible"=w702) -> ()  [unwired: 2 in, 2 out]
        n308 = property on="Motor_Sel (Round)" class="Bool (strict)"("Visible"=w702) -> ()  [unwired: 2 in, 2 out]
        n309 = property on="Motor_Sel (Square)" class="Bool (strict)"("Visible"=w702) -> ()  [unwired: 2 in, 2 out]
        n310 = property on="Alarm Pop-up" class="TabCtl (strict)"("Visible"=w702) -> ()  [unwired: 2 in, 2 out]
        n311 = property on="Info Pop-up" class="TabCtl (strict)"("Visible"=w702) -> ()  [unwired: 2 in, 2 out]
        n312 = property on="Settings Pop-up" class="TabCtl (strict)"("Visible"=w702) -> ()  [unwired: 2 in, 2 out]
        n313 = property on="Main Tab" class="TabCtl (strict)"("DisabledEnum"=w698) -> ()  [unwired: 2 in, 2 out]
        n314 = Bundle By Name(cluster=w700, "Active Alarm"=w701, "Params Open"=w701) -> (w703:T20)
        n315 = Insert Into Array(array=w705, index=0, new element=string[] []) -> (w704:string[])
      }
      frame "Motor/VFD Toggle" {
        n316 = Unbundle By Name(w711) -> ("debug"=w708:bool, "Pop-up Config.Motor/VFD"=w710:T16, "Motor Toggle"=w709:bool)
        n317 = case shown="False" w708 {
          tunnel: w710 -> [w719 _]
          tunnel: w709 -> [w717 _]
          frame False {
            n318 = case shown="\"U-Trough\"" w719 {
              tunnel: [HMI_Coils."MC100_HMI_WS_Drag_PB" ("HMI Coil") HMI_Coils."MC101_HMI_WB_Drag_PB" ("HMI Coil") HMI_Coils."MC102_HMI_WS_Fan_PB" ("HMI Coil") HMI_Coils."MC103_HMI_WB_Fan_PB" ("HMI Coil") HMI_Coils."MC104_HMI_Dryr_Drag_PB" ("HMI Coil") HMI_Coils."MC105_HMI_Dryr_Fan_PB" ("HMI Coil") HMI_Coils."MC106_HMI_DB_Fan_PB" ("HMI Coil") HMI_Coils."MC107_HMI_DB_Drag_PB" ("HMI Coil") HMI_Coils."MC108_HMI_DB_Top_Feed_PB" ("HMI Coil") HMI_Coils."MC109_HMI_U-Trough_PB" ("HMI Coil") HMI_Coils."MC110_HMI_Leg_PB" ("HMI Coil")] -> w718
              frame "WS_Drag", Default {
              }
              frame "WB_Drag" {
              }
              frame "WS_Fan" {
              }
              frame "WB_Fan" {
              }
              frame "Dryer_Drag" {
              }
              frame "Dryer_Fan" {
              }
              frame "DB_Fan" {
              }
              frame "DB_Drag" {
              }
              frame "DB_Top_Feed" {
              }
              frame "U-Trough" {
              }
              frame "Leg" {
              }
            }
            n319 = call "Modbus Global.vi"("HMI Coil"=w718, "Modbus Mode (Write Coil)"=Modbus_Mode."Write Coil", "Coil IN"=w717) -> ()  [unwired: 9 in, 4 out]
          }
          frame True {
          }
        }
        n320 = Insert Into Array(array=w713, index=0, new element=string[] []) -> (w712:string[])
      }
      frame "Send VFD CMD" {
        n321 = Unbundle By Name(w734) -> ("debug"=w731:bool, "Pop-up Config.Motor/VFD"=w733:T16, "VFD_CMD"=w732:dbl)
        n322 = case shown="False" w731 {
          tunnel: w733 -> [w743 _]
          tunnel: w732 -> [w741 _]
          frame False {
            n323 = local write "VFD_CMD"(w741) -> ()
            n324 = Multiply(x=w741, y=100.0) -> (x*y=w740:dbl)
            n325 = case shown="\"U-Trough\"" w743 {
              tunnel: [HMI_Registers."MHR100_HMI_DB_Fan_CMD" ("HMI Reg") HMI_Registers."MHR101_HMI_DB_Drag_CMD" ("HMI Reg") HMI_Registers."MHR102_HMI_DB_TF_CMD" ("HMI Reg") HMI_Registers."MHR103_HMI_U_Trough_CMD" ("HMI Reg") HMI_Registers."MHR104_HMI_Leg_CMD" ("HMI Reg")] -> w742
              frame "DB_Fan", Default {
              }
              frame "DB_Drag" {
              }
              frame "DB_Top_Feed" {
              }
              frame "U-Trough" {
              }
              frame "Leg" {
              }
            }
            n326 = To Unsigned Word Integer(number=w740) -> (unsigned 16bit integer=w739:u16)
            n327 = call "Modbus Global.vi"("Modbus Mode (Write Coil)"=Modbus_Mode."Write Reg", "HMI Reg"=w742, "Reg Data IN"=w739) -> ()  [unwired: 9 in, 4 out]
          }
          frame True {
          }
        }
        n328 = Insert Into Array(array=w736, index=0, new element=string[] []) -> (w735:string[])
      }
      frame "Mode Toggle" {
        n329 = Unbundle By Name(w753) -> ("debug"=w751:bool, "Mode Toggle"=w752:bool)
        n330 = case shown="False" w751 {
          tunnel: w752 -> [w759 _]
          frame False {
            n331 = call "Modbus Global.vi"("HMI Coil"=HMI_Coils."MC121_HMI_Mode_Toggle", "Modbus Mode (Write Coil)"=Modbus_Mode."Write Coil", "Coil IN"=w759) -> ()  [unwired: 9 in, 4 out]
          }
          frame True {
          }
        }
        n332 = Insert Into Array(array=w755, index=0, new element=string[] []) -> (w754:string[])
      }
      frame "Shutdown" {
        # "Turn off all motors."
        n333 = call "Modbus Global.vi"("HMI Coil"=HMI_Coils."MC120_HMI_Shutdown", "Modbus Mode (Write Coil)"=Modbus_Mode."Write Coil", "Coil IN"=TRUE) -> ()  [unwired: 9 in, 4 out]
        n334 = Insert Into Array(array=w766, index=0, new element=string[] []) -> (w765:string[])
      }
      frame "Exit" {
        n335 = Unbundle By Name(w771) -> ("Connected"=w770:bool)
        n336 = property class="App"() -> ("App.Kind"=w769:T31)  [unwired: 2 in, 2 out]
        n337 = case shown="\"Run Time System\"" w769 {
          frame Default {
          }
          frame "Run Time System" {
            n338 = control-ref of="This VI"() -> (w777:refnum<vi>)
            n339 = invoke class="VI" method="FP.Close"(reference=w777) -> ()  [unwired: 2 in, 3 out]
          }
        }
        n340 = case shown="True" w770 {
          frame False {
          }
          frame True {
            n341 = call "Modbus Global.vi"("Modbus Mode (Write Coil)"=Modbus_Mode."Close" ("Modbus Mode")) -> ()  [unwired: 11 in, 4 out]
          }
        }
        n342 = Insert Into Array(array=w774, index=0, new element=string[] []) -> (w773:string[])
        "Loop Stop" <- TRUE ("Modbus Stop")
      }
    }
  }
  n343 = case shown="False" "debug" {
    tunnel: w24 -> [w783 _]
    tunnel: TRUE ("status") -> [w782 _]
    tunnel: w13 -> [w781 _]
    tunnel: w7 -> [w780 _]
    tunnel: w3 -> [w779 _]
    tunnel: w2 -> [_ _]
    frame False {
      n344 = while {
        tunnel: w780 -> [_]
        shift-right: [w807] -> _
        shift-left: w783 -> [w808]
        shift-right: [w801] -> _
        shift-left: w782 -> [w800]
        stop <- w810 stop-if-true
        n345 = Wait (ms)(milliseconds to wait=u32 50) -> ()  [unwired: 1 out]
        n346 = case shown="True" w800 {
          tunnel: [errorcluster {"status"=FALSE, "code"=0, "source"=""} ("Error OUT") w812] -> w805
          frame False {
          }
          frame True {
            n347 = call "Modbus Global.vi"("Modbus Mode (Write Coil)"=Modbus_Mode."Init" ("Modbus Mode")) -> ("Error OUT"=w812:errorcluster)  [unwired: 11 in, 3 out]
          }
        }
        n348 = local read "Heartbeat IN"() -> (w799:bool)
        n349 = Not(x=w808) -> (.not. x?=w807:bool)
        n350 = Not(x=w799) -> (.not. x?=→"Heartbeat OUT":bool)
        n351 = call "Modbus Global.vi"("Modbus Mode (Write Coil)"=Modbus_Mode."Read" ("Modbus Mode"), "Error IN"=w805) -> ("Coils OUT"=→"Coils OUT":bool[], "Registers OUT"=→"Registers OUT":u16[], "Error OUT"=w802:errorcluster)  [unwired: 10 in, 1 out]
        n352 = Unbundle By Name(w802) -> ("status"=w801:bool)
        n353 = local read "Loop Stop"() -> (w810:bool)
      }
      n354 = while {
        tunnel: w781 -> [w797]
        tunnel: w780 -> [_]
        tunnel: w779 -> [_]
        stop <- w793 stop-if-true
        n355 = local read "Bin Levels"() -> (w790:u16[])
        n356 = local read "Auto Mode"() -> (w785:bool)
        n357 = Index Array(array=w790) -> (element #1=w789:u16, element #2=w788:u16, element #3=w787:u16, element #4=w786:u16)  [unwired: 4 in]
        n358 = Boolean To (0,1)(Boolean=w785) -> (0, 1=w784:i16)
        n359 = Format Into String(format string="{\n\t\"dry_bin_level\": %d,\n\t\"dryer_bin_level\": %d,\n\t\"wet_bin_level\": %d,\n\t\"wet_silo_level\": %d,\n\t\"auto_mode\": %d\n}" ("buffer"), w789, w788, w787, w786, w784) -> (resulting string=w794:string)  [unwired: 2 in, 1 out]
        n360 = call-poly <vilib>:"POST.vi"("client handle"=w797, "url"=" https://tetilengineering.aws.thinger.io/v3/users/gtetil/devices/swoishGrain/callback/data", "buffer"=w794) -> ("error out"=w791:errorcluster)  [unwired: 9 in, 3 out]
        n361 = Wait (ms)(milliseconds to wait=u32 1000) -> ()  [unwired: 1 out]
        n362 = call <vilib>:"Clear Errors.vi"("error in (no error)"=w791) -> ()  [unwired: 5 in, 2 out]
        n363 = local read "Loop Stop"() -> (w793:bool)
      }
      n364 = while {
        tunnel: w780 -> [_]
        stop <- w818 stop-if-true
        n365 = call "Email Global.vi"() -> ("Emails OUT"=w814:T9[], "Message OUT"=w815:string, "Send Email"=w816:bool)  [unwired: 9 in]
        n366 = Wait (ms)(milliseconds to wait=u32 1000) -> ()  [unwired: 1 out]
        n367 = case shown="True" w816 {
          tunnel: w815 -> [_ w820]
          tunnel: w814 -> [_ w819]
          frame False {
          }
          frame True {
            n368 = for {
              tunnel: w820 -> [w824]
              tunnel: w819 -> [w823] mode=indexing
              n369 = Unbundle By Name(w823) -> ("Email"=w821:string, "Enabled"=w822:bool)
              n370 = case shown="True" w822 {
                tunnel: w824 -> [_ w826]
                tunnel: w821 -> [_ w825]
                frame False {
                }
                frame True {
                  n371 = call "Python Email.vi"("To:"=w825, "Message:"=w826) -> ()  [unwired: 9 in, 5 out]
                }
              }
            }
          }
        }
        n372 = local read "Loop Stop"() -> (w818:bool)
      }
    }
    frame True {
    }
  }
